vi "UHR-Fleezers Control (fpga) - Leonardo 04-2018.vi"() -> ()   [LabVIEW 2013]
doc: "UHR-Fleezers Instrument Control Code (fpga)"
uses:
  <vilib>/Platform/TimedLoop/XDataNode/timing_clust.ctl
  <vilib>/Platform/TimedLoop/XDataNode/nitl_modes.ctl
  <vilib>/Platform/TimedLoop/XDataNode/wakeup.ctl
  <vilib>/rvi/eio/common/nirviEmuTemplateMethod_errors.vi
  <vilib>/rvi/Emulation/niFpgaSctlEmulationGetInTimedLoop.vi
  <vilib>/rvi/Emulation/niFpgaEmulationReportErrorSimple.vi
  <vilib>/rvi/Emulation/niFpgaGetClockAttributes.vi
  <vilib>/rvi/Emulation/niFpgaCriticalErrorInLSC.vi
  <vilib>/rvi/FIFO/Fifo_Resource/nirvififoEmulationReadFpgaImpl.vi
  <vilib>/rvi/DataTransferAndStorage/Container/Common/niFpgaContainerGetUniqueNameForEmu.vi
  <vilib>/rvi/DataTransferAndStorage/Container/Common/niFpgaContainerExecOnDevCompGetState.vi
  <vilib>/rvi/interface/RandomDataEmulation/nirviRandomDataFPGAFIFO.vi
  <vilib>/rvi/interface/RandomDataEmulation/niFpgaRandomDataHandleErrors.vi
  <vilib>/rvi/eio/common/nirviEmuReportErrorAndStop.vi
  <vilib>/rvi/Emulation/niFpgaProcessEmulError.vi
  <vilib>/rvi/FIFO/Fifo_Resource/nirvififoEmulationWriteFpgaImpl.vi
  <vilib>/rvi/Memory/Memory_Emulation/nirvimemoryFastEmulationFpgaImpl.vi
  <instcachedir>/0/nirvimemoryFastEmulationFpgaImpl_5FBAB50466BC4C939F684F8805638BFC.lvgen/nirvimemoryFastEmulationFpgaImpl_5FBAB50466BC4C939F684F8805638BFC_002.vi
  <vilib>/rvi/Memory/Memory_Emulation/niFpgaMemoryEmulationCacheClearOnFirstRun.vi
  <vilib>/rvi/Memory/Memory_Emulation/nirvimemoryEmulationManagerCache_MakeExclusive.vi
  <vilib>/rvi/Memory/Memory_Emulation/niFpgaMemoryEmulationValidateCache.vi
  <vilib>/rvi/Memory/Memory_Emulation/nirvimemoryEmulationManagerCache_ReleaseExclusive.vi
  <vilib>/rvi/Memory/Memory_Emulation/nirvimemoryEmulationManagerCache_InsertValue.vi
  <vilib>/Utility/error.llb/Clear Errors.vi
  <vilib>/rvi/Memory/Memory_Emulation/nirvimemoryEmulationManagerCache_GetValue.vi
  <vilib>/Platform/TimedLoop/XDataNode/XDataNode.xnode
  <vilib>/eio/EIOMethodNode/EIOMethodNode.xnode
  <vilib>/eio/EIONode/EIONode.xnode
  <vilib>/rvi/DataTransferAndStorage/Container/XNode/niFpgaContainer.xnode
  <vilib>/rvi/FIFO/Fifo_Resource/nirvififoEmulationRead.vi
  <vilib>/rvi/FIFO/Fifo_Resource/niFpgaFifoEmulationRefIn.vi
  <vilib>/rvi/interface/RandomDataEmulation/nirviRandomDataFpgaReadWriteTemplate.vi
  <vilib>/rvi/FIFO/Fifo_Resource/nirvififoEmulationWrite.vi
  <vilib>/rvi/Memory/Memory_Emulation/niFpgaMemoryEmulationRefIn.vi
  <vilib>/addons/control/pid/fpga.llb/XNode/niFpgaPID.xnode
  <vilib>/Platform/TimedLoop/XDataNode/XDNodeRunTimeDep.lvlib
panel:
  in  "Tab Control 2":T1(tab)
  out "BD1 amplitude 1 out":u16
  out "BD1 amplitude 2 out":u16
  in  "FB output range":cluster{"output low":i16, "output high":i16}={"output low"=0, "output high"=3000}
  in  "FB Gains":T2={"proportional gain (Kc)"=10, "integral gain (Kc*Ts/Ti)"=5, "derivative gain (Kc*Td/Ts)"=0}
  in  "RF synth green feedback max":i16=4000
  in  "RD":bool=TRUE
  in  "Swap F1 and F2":bool
  in  "Cont. Scan":bool
  in  "Abort scan":bool
  in  "Cycles per step":u64
  in  "Scan BD":bool
  in  "Number of scans":u16
  in  "Scan steps":u64
  in  "Scan freq.  increment":i64
  out "Scanning":bool
  in  "Start scan":bool
  in  "OSK Bd 1":bool
  in  "Reset Bd 1":bool
  in  "PMODE":bool=TRUE
  in  "Number Interlace Cycles":u8=2 min=1 max=3
  in  "Interlace Off Parameters":u8=1 min=1 max=3
  in  "Interlace ON/OFF":bool
  out "DIO Relative phase":i16
  in  "Phase count adjustment (DIO)":i16
  in  "+ phase (DIO)":bool
  out "DIO Late Counter":u8
  in  "DIO count 1 (ticks)":u16=400
  in  "DIO count 2 (ticks)":u16=400
  in  "DIO count 3 (ticks)":u16=400
  out "AI2 Y Sum Set 2":i16
  out "AI2 Y Sum Set 1":i16
  in  "FB Setpoint Set 1":i16 min=0 step=1
  in  "FB Reset Set 1":bool
  in  "FB On/Off Set 1":bool
  in  "FB Reset Set 2":bool
  in  "FB On/Off Set 2":bool
  in  "FB Setpoint Set 2":i16 min=0 step=1
  out "Scan I":u64
  in  "Amp switch delay":u8=5
  in  "RF synth bd controls green":bool
  in  "Phase Trap 2":fxp<+,14,14>
  in  "Phase Trap 1":fxp<+,14,14>
  in  "Phase offset method":u8
  in  "BD 2 Amplitude 1":u16
  in  "BD 1 Amplitude 1":u16
  in  "BD 2 Frequency 1":u64
  in  "BD 1 Frequency 1":u64
  in  "BD 2 Amplitude 2":u16
  in  "BD 1 Amplitude 2":u16
  in  "BD 2 Frequency 2":u64
  in  "BD 1 Frequency 2":u64
  in  "BD 2 Amplitude 3":u16
  in  "BD 1 Amplitude 3":u16
  in  "BD 2 Frequency 3":u64
  in  "BD 1 Frequency 3":u64
  in  "BD 2 Delay (Ticks)":u8 caption="Count(Ticks)"
  in  "Next trap write delay (ticks)":u8 caption="Count(Ticks)"
  out "Random phase generated":fxp<+,14,14>
  in  "RF phase reset before cycles":bool
  in  "Trap 1 osc enable":bool
  in  "N trap osc periods":i16
  in  "Trap osc period (pts)":i16
  in  "Osc traps":bool
  in  "Initiate trap osc":bool
  in  "Ready Write":bool
  in  "Data":i64
  in  "Address 2":u32
  in  "Osc trap cont.":bool
  in  "Trap 2 osc enable":bool
  out "green FB running":bool
  in  "APD 2 AO scale factor":i16=1
  in  "BD 1 Delay (ticks)":u8
  in  "Tab Control":T3(tab)=enum."MCL trap control"
  in  "Set 3":bool
  in  "Set 2":bool=TRUE
  in  "Set 1":bool=TRUE
  in  "Trap Pos to FIFO":bool
  in  "N of AI1 Int Acq Sets":i16=2 min=1 max=3 step=1
  out "AI Late Counter":u8
  in  "ai count":u16=400
  in  "+ phase":bool
  in  "Phase count adjustment":i16
  out "Relative phase":i16
  in  "AI to FIFO":bool
  out "BD1 Frequency Out 1":u64
  out "BD1 Frequency Out 2":u64
  out "Trap Pos FIFO Timeout":u16
  out "Trap AI FIFO Timeout":u16
  in  "Trap FIFO Set Timeout":i32
  in  "FB Min frequency":u64
  in  "FB Max Frequency":u64
  in  "Dynamic Force FB (Ronen)":bool
  in  "Trap pos. FB Range":T4={"FB2 output low"=-1.0, "FB2 output high"=0.999969482421875}
  in  "Trap Pos. FB Gains":T5={"proportional gain (Kc)"=0.999969482421875, "integral gain (Kc*Ts/Ti)"=0.999969482421875, "derivative gain (Kc*Td/Ts)"=0.0}
  in  "B factor":fxp<+/-,32,16>
  in  "Negate Diff?":bool
  in  "Diff FB Measurement?":bool
  in  "FB Trig Integrate":u32=1
  out "TTrig?":bool
  in  "TTrig Negate Pos":bool=TRUE
  out "Trap Pos FB Int Signal":fxp<+/-,24,9> format="%.18g"
  out "Trap Pos FB Int-Norm Signal":fxp<+/-,16,1> format="%.16g"
  in  "FPGA TTrig Thresh":i64
  in  "FPGA Trap Trig":bool
  out "Trap Pos FB Action":i64
  in  "Trap Pos. FB Offset Factor":i64
  in  "Trap Pos. FB Mult Factor":i64=2
  in  "Trap Pos. FB Reset":bool
  in  "Trap Pos FB Monitor T1 or T2":bool
  in  "AI1 X Scale":u16
  in  "Trap Pos FB Int Count":u16=100
  in  "Trap Pos FB Negate Action":bool
  out "AI1 X Set 2":fxp<+/-,16,1>
  out "AI1 X Set 1":fxp<+/-,16,1>
  in  "Trap Pos. FB SP":fxp<+/-,16,1>
  in  "Force feedback":bool
  out "TTrig Sig":i64
  out "TTrig Fin Thresh":i64
  in  "1D or 2D Scan?":bool
  in  "Abort scan (MCL)":bool
  in  "MCL Scan Axis":bool
  in  "Cont. Scan (MCL)":bool
  out "Scan I (MCL)":u64
  in  "Number of scans (MCL)":u16
  out "Scanning MCL":bool
  in  "Scan steps (MCL)":u64
  in  "Cycles per step (MCL)":u64
  in  "Scan freq.  increment (MCL)":i16
  in  "Start scan (MCL)":bool
  in  "AO2 (X)":i16
  in  "AO1 (Y)":i16
  out "MCL Late Counter":u8
  in  "MCL count":u32=800
  out "MCL Relative Phase":i16
  in  "Phase count adjustment (MCL)":i16
  in  "+ phase (MCL)":bool
  in  "Lifetime events to read blue":u16=100
  in  "Lifetime read blue fifo":bool
  out "lifetime events in fifo":u16
  out "APD2 int gate":bool
  in  "APD Gate Operating Mode":u8 max=2 step=1
  in  "Invert APD Gate":bool
  in  "APD Gate OFF Count":u16=100
  in  "APD Gate ON Count":u16=300
  out "APD 1 Gate Late Counter":u8
  out "APD 1 Gate Relative Phase":i16
  in  "Phase count adjustment (APD 1 Gate)":i16
  in  "+ phase (APD 1 Gate)":bool
  out "APD 2 Counts 0":u32
  out "APD 2 Counts 1":u32
  out "APD 1 Counts 0":u32
  out "APD 1 Counts 1":u32
  in  "Phase count adjustment (APD 2 Gate)":i16
  out "APD 2 Gate Late Counter":u8
  out "APD 2 Gate Relative Phase":i16
  in  "+ phase (APD 2 Gate)":bool
  out "APD 3 Counts 0":u32
  out "APD 3 Counts 1":u32
  out "APD 3 Gate Late Counter":u8
  in  "Phase count adjustment (APD 3 Gate)":i16
  out "APD 3 Gate Relative Phase":i16
  in  "+ phase (APD 3 Gate)":bool
  out "APD1 int gate":bool
  out "APD3 int gate":bool
  in  "Lifetime timeout APD1":u16=200
  in  "APD to FIFO":bool
  in  "APD Acq Rate Count":u32=20000000
  out "APD Acq Late Counter":u16
  out "APD Acq Relative Phase":i16
  in  "+ phase (APD Acq)":bool
  in  "Phase Count Adjustment (APD Acq)":i16
  in  "APD 1 AO scale factor":i16=1
  out "APD2 out state":bool
  out "APD1 out state":bool
  out "APD Acq Late?":bool
  in  "D3 2":i16
  in  "I3 2":i16=5
  in  "P3 2":i16=10
  in  "Green FB Setpoint 2":i16=250 min=0 step=1
  in  "Green FB Reset 2":bool
  in  "Green Filter Flipper":bool
  in  "Green interlace OFF count":u16=100
  out "GI Relative phase":i16
  in  "Phase count adjustment (GI)":i16
  in  "+ phase (GI)":bool
  in  "Green interlace ON count":u16=300
  out "GI Late Counter":u8
  in  "Invert GI":bool
  in  "Operating Mode":u8 max=2 step=1
  in  "Current Out":u16=30000
  in  "Green int current ON count adj":u32=150
  in  "Green interlace OFF count":u32=900
  in  "Green interlace ON count":u32=300
  out "GI Late Counter":u16
  in  "Green FB Count":u32=1200
  in  "Phase count adjustment (GI)":i16=20
  in  "Green FB Setpoint":i16=250 min=0 step=1
  in  "Invert GI":bool
  out "GI Relative phase":i16
  in  "+ phase (GI)":bool
  in  "Phase count adjustment (Green FB)":i16=10
  out "Green Late Counter":u16
  out "Green FB Relative Phase":i16
  in  "+ phase (Green FB)":bool
  out "Green FB Signals":T6
  out "Green FB Sum":i16
  in  "Green FB Gains":T2={"proportional gain (Kc)"=10, "integral gain (Kc*Ts/Ti)"=5, "derivative gain (Kc*Td/Ts)"=0}
  in  "Green FB On/Off":bool
  in  "Green FB Reset":bool
  out "Green FB Late?":bool
  out "GI Late?":bool
  in  "Operating Mode 2":u8=2 max=2 step=1
  in  "+ phase (RI)":bool
  out "RI Relative phase":i16
  out "RI Late Counter":u8
  in  "Red interlace ON count":u16=300
  in  "Red interlace OFF count":u16=100
  in  "Invert RI":bool
  in  "Red Laser Operating Mode":u8 max=2 step=1
  in  "Phase count adjustment (RI)":i16
  in  "Phase count adjustment (BI D)":i16
  in  "Blue Laser Operating Mode (D)":u8 max=2 step=1
  in  "Invert BI (D)":bool
  in  "Blue interlace OFF count (D)":u16=100
  in  "Blue interlace ON count (D)":u16=300
  out "Blue Late Counter (D)":u8
  out "BI Relative phase (D)":i16
  in  "+ phase (BI D)":bool
  in  "Lifetime to FIFO":bool
  out "lifetime (ticks)":u16
  # "Raster Scan AOD"
  # "1 (X)"
  # "2 (Y)"
  # "IR Intensity Feedback (RF BD 1)"
  # "FB Gains Set 1"
  # "FB output range 1"
  # "IR Intensity Feedback (RF BD 2) -\nonly when using BD 2 for green laser AOM (not trap Y)"
  # "Keep below 4096 (12 bits) to stay within range of RF board. Going over doesn't saturate, it truncates higher bits."
  # "RF phase offset control"
  # "Methods are:\n0 - Default, do nothing at all (no phase offset writes)\n1 - Manual phase adjustment\n2 - Cycle the phase adjustment using the input phase numbers as increment values for each cycle"
  # "False is usual, True is external loop method"
  # "Parameters if using the external RF switching loop"
  # "Parameters if using the usual internal RF switching method"
  # "FB Triggering Excitation Laser"
  # "Trap Pos. FB Gains"
  # "Trap Pos. FB Range"
  # "AO1 (Y)"
  # "2D"
  # "Trap 3"
  # "1D"
  # "AO2 (X)"
  # "Fl Laser"
  # "APD AO for aligning"
  # "Detection Loop"
  # "Green fluorescent laser digital gate interlacing loop"
  # "0 Forced ON\n1 Forced OFF\n2 Interlacing"
  # "ALEX settings:"
  # "Controls for usual IA ME controls green AOM"
  # "Controls for RF synth board controls green AOM"
  # "Green FB Gains"
  # "Red fluorescent laser digital gate interlacing loop"
  # "Detection Loop"
  # "0 Forced ON\n1 Forced OFF\n2 Interlacing"
  # "Analog/FB Control Loop\n(Disabled)"
  # "Digital Control Loop"
  # "Blue laser intensity reading"
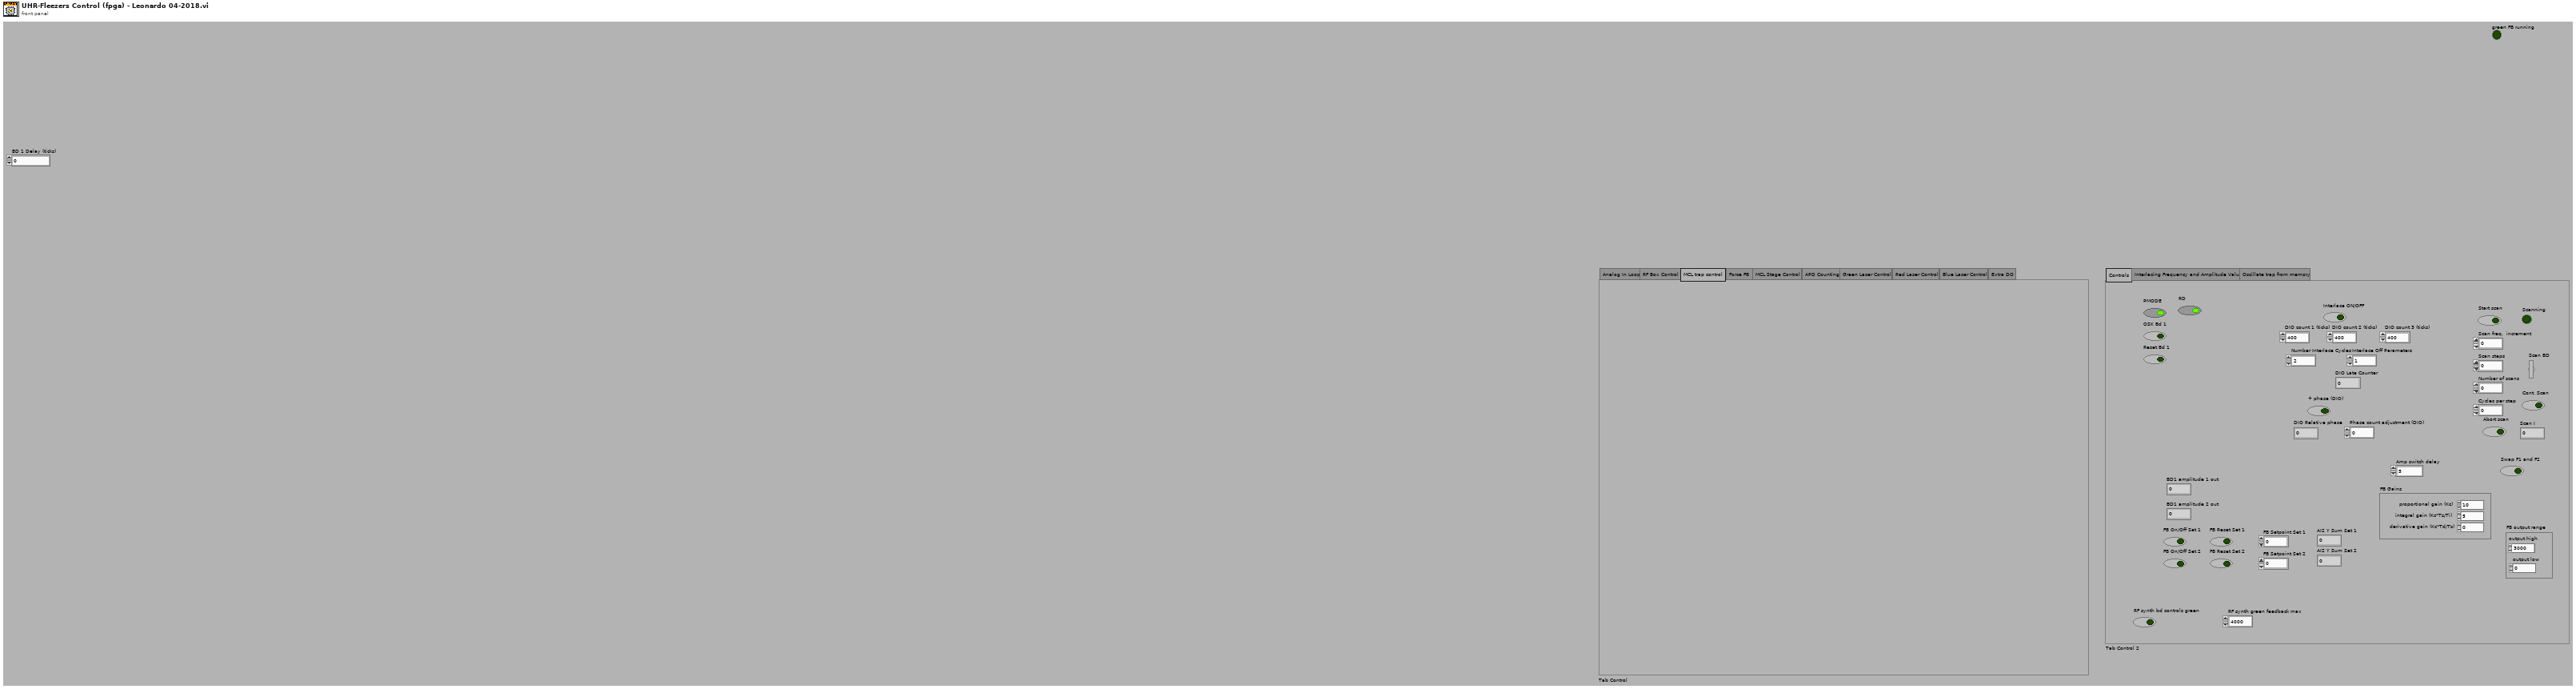
[diagram p1: front panel]
types:
  T1 = enum32{"Controls", "Interlacing Frequency and Amplitude Values", "Oscillate trap from memory"}
  T2 = cluster{"proportional gain (Kc)":i16, "integral gain (Kc*Ts/Ti)":i16, "derivative gain (Kc*Td/Ts)":i16}
  T3 = enum32{"Analog In Loop", "RF Box Control", "MCL trap control", "Force FB", "MCL Stage Control", "APD Counting", "Green Laser Control", "Red Laser Control", "Blue Laser Control", "Extra DO"}
  T4 = cluster{"FB2 output low":fxp<+/-,16,1>, "FB2 output high":fxp<+/-,16,1>}
  T5 = cluster{"proportional gain (Kc)":fxp<+/-,16,1>, "integral gain (Kc*Ts/Ti)":fxp<+/-,16,1>, "derivative gain (Kc*Td/Ts)":fxp<+/-,16,1>}
  T6 = cluster{"Green FB Ch 0":i16, "Green FB Ch 1":i16, "Green FB Ch 2":i16}
  T7 = typedef "XDNodeRunTimeDep.lvlib/timing_clust.ctl" = cluster{"Expected End [f-1]":u64, "Actual End [f-1]":u64, "Finished Late? [f-1]":bool, "Expected End [i-1]":u64, "Actual End [i-1]":u64, "Finished Late? [i-1]":bool, "Expected Start [i]":u64, "Actual Start [i]":u64, "Expected Start [f]":u64, "Actual Start [f]":u64, "Source Name":string, "Structure Name":string, "Period":i64, "Deadline":i64, "Offset":i64, "Start":i64, "Priority":i32, "Timeout":i32, "Mode":T8, "Wakeup Reason":T9, "Error":errorcluster, "Source Type":string, "Secondary Source Type":string, "Global End Time":u64, "Global Start Time":u64, "Frame Duration":u64, "Iteration Duration":u64, "Assigned CPU":i32, "I/O Scan Engine Mode":u32}
  T8 = typedef "XDNodeRunTimeDep.lvlib/nitl_modes.ctl" = enum32{"No Change", "Process missed periods, maintain original phase", "Discard missed periods, maintain original phase", "Process missed periods, ignore original phase", "Discard missed periods, ignore original phase"}
  T9 = typedef "XDNodeRunTimeDep.lvlib/wakeup.ctl" = enum32{"Normal", "Aborted", "Asynchronous wakeup", "Timing source error", "Timed loop error", "Timeout"}
  T10 = cluster{"Chassis2/Mod2/AI0":i16, "Chassis2/Mod2/AI1":i16, "Chassis2/Mod2/AI2":i16}
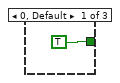
[diagram p3: hidden frame]
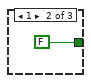
[diagram p4: hidden frame]
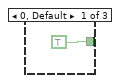
[diagram p8: hidden frame]
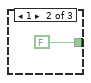
[diagram p9: hidden frame]
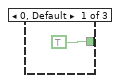
[diagram p10: hidden frame]
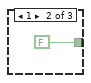
[diagram p11: hidden frame]
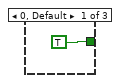
[diagram p13: hidden frame]
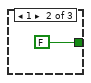
[diagram p14: hidden frame]
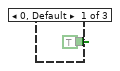
[diagram p15: hidden frame]
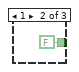
[diagram p16: hidden frame]
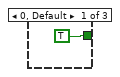
[diagram p18: hidden frame]
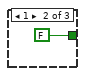
[diagram p19: hidden frame]
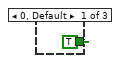
[diagram p20: hidden frame]
diagram:
  w3 = FALSE
  w4 = FALSE
  # "BD2 amp"
  # "BD1 amp"
  # "BD2 amp"
  # "BD1 amp"
  # "timing array current index"
  # "timing array"
  # "timing counter (phase adjusted here)"
  # "late counter"
  n1 = disable-structure shown="Disabled" {
    frame Disabled {
      w14 = i16 2 items=["UnSet Ready", "ReadWrite", "Wait Ready"]
      n2 = while "Handshake memory transfer for trap oscillation sin wave data" {
        shift-right: [w16] -> _
        shift-left: w14 -> [w17]
        stop <- FALSE stop-if-true
        # "Write"
        n3 = case shown="1" w17 {
          tunnel: [w20 w25 w26] -> w16
          frame 3, Default {
            w18 = i16 2 items=["UnSet Ready", "ReadWrite", "Wait Ready"]
            w19 = i16 1 items=["UnSet Ready", "ReadWrite", "Wait Ready"]
            n4 = Select(t=w19, s="Ready Write", f=w18) -> (s? t:f=w20:i16)
          }
          frame 1 {
            w25 = i16 0 items=["UnSet Ready", "ReadWrite", "Wait Ready"]
            n5 = xnode ("Memory Write")("Address"="Address 2", "Data"="Data", "Memory In"=refnum<k21> "Trap osc memory") -> ()  [unwired: 1 out]
          }
          frame 0 {
            w26 = i16 2 items=["UnSet Ready", "ReadWrite", "Wait Ready"]
            n6 = local write "Ready Write"(FALSE ("Ready Read")) -> ()
          }
        }
      }
    }
    frame Enabled {
    }
  }
  n7 = flat-sequence "FPGA initialization to do before running any of the loops" {
    tunnel: [u16 0 ("DIO count 3 (ticks)")] -> w2
    tunnel: [w35] -> _
    frame #0 {
      # "UDCLK out enable and set low"
      # "WR"
      # "BD 2"
      # "BD 1"
      # "With the RF synth board initialization now done in a separate fpga vi, now when this vi is started, board is already configured and is ready for interlacing. Just need to set WR high and enabled UDCLK as write and set to low.\nbefore setting data and address bits."
      # "Start up expansion chassis early\nto avoid delays later"
      # "Set data and address values to something safe (a correct setting) so any initial WR and udclk flipping doesn't have a chance to mess anything up. Safe would be setting an unused data entry:"
      n8 = xnode "FPGA I/O Method Node"("Enable"=TRUE) -> ("FPGA I/O Out"=w29:refnum<k21>)  [unwired: 1 in]
      n9 = xnode "FPGA I/O Method Node"("Enable"=TRUE) -> ("FPGA I/O Out"=w32:refnum<k21>)  [unwired: 1 in]
      n10 = xnode "FPGA I/O Node"("Chassis2/Mod1/AO0"=u16 0 ("Chassis2/Mod4/AO0")) -> ("Chassis2/Mod2/AI0"=w35:i16)  [unwired: 2 in, 2 out]
      n11 = xnode "FPGA I/O Node"("Connector1/DIO15"=TRUE) -> ()  [unwired: 1 in, 1 out]
      n12 = xnode "FPGA I/O Node"("I/O Item"=FALSE ("Connector1/DIO30"), "FPGA I/O In"=w29) -> ()  [unwired: 1 out]
      n13 = xnode "FPGA I/O Node"("I/O Item"=FALSE ("Connector1/DIO30"), "FPGA I/O In"=w32) -> ()  [unwired: 1 out]
      n14 = xnode "FPGA I/O Node"("Connector1/DIO0"=FALSE, "Connector1/DIO1"=FALSE, "Connector1/DIO2"=FALSE, "Connector1/DIO3"=FALSE, "Connector1/DIO4"=FALSE, "Connector1/DIO5"=FALSE, "Connector1/DIO6"=FALSE, "Connector1/DIO7"=FALSE, "Connector1/DIO8"=FALSE, "Connector1/DIO9"=FALSE, "Connector1/DIO10"=FALSE, "Connector1/DIO11"=FALSE, "Connector1/DIO12"=FALSE, "Connector1/DIO13"=FALSE, "Connector1/DIO20"=FALSE, "Connector1/DIO21"=FALSE, "Connector1/DIO22"=FALSE, "Connector1/DIO23"=FALSE, "Connector1/DIO24"=FALSE, "Connector1/DIO25"=FALSE, "Connector1/DIO26"=FALSE, "Connector1/DIO27"=FALSE, "Connector1/DIO14"=FALSE) -> ()  [unwired: 23 in, 23 out]
    }
  }
  n15 = node-c288() -> (w10:T7)  [unwired: 1 in]
  n16 = timed-loop "RF box board DIO control: control bits" {
    timing: w10 -> [_]
    timing-out: [_] -> w9
    tunnel: [w63] -> _
    tunnel: w2 -> [w63]
    stop <- FALSE stop-if-true
    n17 = xnode "FPGA I/O Node"("Connector1/DIO16"="RD", "Connector1/DIO17"="PMODE", "Connector1/DIO18"="OSK Bd 1", "Connector1/DIO19"="Reset Bd 1", "Connector0/DIO3"="Green Filter Flipper") -> ()  [unwired: 5 in, 5 out]
  }
  n18 = node-c288(w9) -> ()
  n19 = local read "AO1 (Y)"() -> (w12:i16)
  n20 = local read "AO2 (X)"() -> (w11:i16)
  n21 = To Unsigned Long Integer(number=w2) -> (unsigned 32bit integer=w5:u32)
  n22 = while "DAQ AI set 1" {
    shift-right: [w70] -> _
    shift-left: w2 -> [w75]
    stop <- FALSE stop-if-true
    n23 = flat-sequence {
      tunnel: w75 -> [w86]
      tunnel: [w85] -> w73
      tunnel: [w86] -> w72
      tunnel: [w96] -> w83
      tunnel: [w95] -> w82
      tunnel: [w94] -> w81
      tunnel: [w93] -> w80
      tunnel: [w92] -> w79
      tunnel: [w91] -> w78
      tunnel: [w90] -> w77
      tunnel: [w89] -> w76
      tunnel: [w88] -> w74
      tunnel: w73 -> [w88]
      tunnel: w72 -> [w87]
      tunnel: [w87] -> w71
      tunnel: [w126] -> w70
      tunnel: w83 -> [w152]
      tunnel: w82 -> [w118]
      tunnel: w81 -> [w119]
      tunnel: w80 -> [w98]
      tunnel: w79 -> [w142]
      tunnel: w78 -> [w141]
      tunnel: w77 -> [w140]
      tunnel: w76 -> [w139]
      tunnel: w74 -> [w136]
      tunnel: w71 -> [w133]
      frame #0 {
        n24 = call "Loop Timer"("Count(Ticks)"=w86) -> ("Tick Count(Ticks)"=w85:u32)
      }
      frame #1 {
        n25 = xnode "FPGA I/O Node"("Connector1/DIO31"=TRUE ("Connector1/DIO33")) -> ("Connector0/AI0"=w96:i16, "Connector0/AI1"=w95:i16, "Connector0/AI2"=w94:i16, "Connector0/AI3"=w93:i16, "Connector0/AI4"=w92:i16, "Connector0/AI5"=w91:i16, "Connector0/AI6"=w90:i16, "Connector0/AI7"=w89:i16)  [unwired: 9 in, 9 out]
      }
      frame #2 {
        w122 = FALSE ("AI to FIFO")
        # "Normalize by trap bead QPD sum, AI3"
        # "Adjust phase after data acquired if button pressed"
        n26 = feedback #1(i16 1) -> (w145:i16)
        n27 = Increment(x=w145) -> (x+1=w151:i16)
        n28 = Scale By Power Of 2(n="AI1 X Scale", x=w118) -> (x*2^n=w116:i16)
        n29 = Greater?(x=w151, y="N of AI1 Int Acq Sets") -> (0:w148:bool)
        n30 = Select(t=i16 1, s=w148, f=w151) -> (s? t:f=w150:i16)
        n31 = feedback-in #1(w150) -> ()
        n32 = Divide(x=w116, y=w98) -> (x/y=w115:fxp<+/-,16,1>)
        n33 = feedback #2(w122) -> (w120:bool)
        n34 = feedback #3(w122) -> (w138:bool)
        n35 = case shown="1, Default" w145 {
          tunnel: w119 -> [w175 w182 _]
          tunnel: ["Set 1" "Set 2" "Set 3"] -> w143
          tunnel: ["AI to FIFO" w184 w189] -> w137
          tunnel: w138 -> [_ w184 w189]
          tunnel: ["Trap Pos to FIFO" w183 w188] -> w121
          tunnel: w120 -> [_ w183 w188]
          tunnel: w115 -> [w174 w181 _]
          tunnel: [w173 w179 FALSE] -> w102
          tunnel: [w172 w180 u64 0 ("BD1 Frequency Out 2")] -> w101
          frame 1, Default {
            n36 = local read "BD1 Frequency Out 1"() -> (w172:u64)
            n37 = Compound Arithmetic op=AND("Trap Pos to FIFO", "Set 1", "AI to FIFO") -> (w173:bool)
            "AI2 Y Sum Set 1" <- w175
            "AI1 X Set 1" <- w174
          }
          frame 2 {
            n38 = local read "BD1 Frequency Out 2"() -> (w180:u64)
            n39 = Compound Arithmetic op=AND(w183, "Set 2", w184) -> (w179:bool)
            "AI2 Y Sum Set 2" <- w182
            "AI1 X Set 2" <- w181
          }
          frame 3 {
          }
        }
        n40 = And(x=w143, y=w137) -> (x .and. y?=w144:bool)
        n41 = case shown="True" w144 {
          tunnel: w152 -> [_ w203]
          tunnel: w118 -> [_ w202]
          tunnel: w119 -> [_ w201]
          tunnel: w98 -> [_ w200]
          tunnel: w142 -> [_ w199]
          tunnel: w141 -> [_ w198]
          tunnel: w140 -> [_ w197]
          tunnel: w139 -> [_ w196]
          tunnel: 0 ("DMA buffer timeout") -> [_ w205]
          frame False {
          }
          frame True {
            n42 = Build Array(w203, w202, w201, w200, w199, w198, w197, w196) -> (w204:i16[])
            n43 = for {
              tunnel: w204 -> [w207] mode=indexing
              tunnel: w205 -> [w208]
              tunnel: [w206] -> w194 mode=indexing
              n44 = xnode ("FIFO Write")("Element"=w207, "Timeout"=w208) -> ("Timed Out?"=w206:bool)  [unwired: 1 in, 1 out]
            }
            n45 = Or Array Elements(Boolean array=w194) -> (logical OR=w191:bool)
            n46 = Boolean To (0,1)(Boolean=w191) -> (0, 1=w193:i16)
            n47 = feedback #4(u16 0) -> (w192:u16)
            n48 = Add(x=w193, y=w192) -> (x+y=w190:u16)
            "Trap AI FIFO Timeout" <- w190
            n49 = feedback-in #4(w190) -> ()
          }
        }
        n50 = feedback-in #2(w121) -> ()
        n51 = feedback-in #3(w137) -> ()
        n52 = case shown="True" w102 {
          tunnel: w101 -> [_ w158]
          tunnel: [u8 0 w155] -> w100
          frame False {
          }
          frame True {
            n53 = Split Number(x=w158) -> (hi(x)=w159:u32, lo(x)=w160:u32)
            n54 = Split Number(x=w159) -> (lo(x)=w161:u16)  [unwired: 1 out]
            n55 = Split Number(x=w160) -> (hi(x)=w162:u16, lo(x)=w163:u16)
            n56 = Build Array "BD 1 nu Stack"(w161, w162, w163) -> (w157:u16[])
            n57 = for {
              tunnel: w157 -> [w170] mode=indexing
              shift-right: [w166] -> w155
              shift-left: u8 0 -> [w167]
              n58 = xnode ("FIFO Method Node")("Element"=w170, "Timeout"="Trap FIFO Set Timeout") -> ("Timed Out?"=w169:bool)  [unwired: 1 in, 1 out]
              n59 = Boolean To (0,1)(Boolean=w169) -> (0, 1=w168:i16)
              n60 = To Unsigned Byte Integer(number=w168) -> (unsigned 8bit integer=w165:u8)
              n61 = Add(x=w165, y=w167) -> (x+y=w166:u8)
            }
          }
        }
        n62 = To Unsigned Word Integer(number=w100) -> (unsigned 16bit integer=w99:u16)
        n63 = feedback #5(u16 0) -> (w113:u16)
        n64 = Add(x=w99, y=w113) -> (x+y=w112:u16)
        "Trap Pos FIFO Timeout" <- w112
        n65 = feedback-in #5(w112) -> ()
        n66 = feedback-in #6(w136) -> ()
        n67 = feedback #6(w136) -> (w135:u32)
        n68 = Subtract(x=w136, y=w135) -> (x-y=w134:u32)
        n69 = xnode "FPGA I/O Node"("Connector1/DIO31"=FALSE ("Connector1/DIO34")) -> ()  [unwired: 1 in, 1 out]
        n70 = Subtract(x=w134, y=w133) -> (x-y=w104:u32)
        n71 = Boolean To (0,1)(Boolean="+ phase") -> (0, 1=w129:i16)
        n72 = Multiply(x=w129, y="Phase count adjustment") -> (x*y=w123:i16)
        n73 = Subtract(x="ai count", y=w104) -> (x-y=w127:u32)
        n74 = Number To Boolean Array(number=w104) -> (Boolean array=w105:bool[])
        n75 = feedback #7(i16 0) -> (w125:i16)
        n76 = Add(x=w127, y=w123) -> (x+y=w126:u32)
        n77 = Subtract(x=w125, y=w123) -> (x-y=w124:i16)
        "Relative phase" <- w124
        n78 = feedback-in #7(w124) -> ()
        n79 = Or Array Elements(Boolean array=w105) -> (logical OR=w103:bool)
        n80 = Boolean To (0,1)(Boolean=w103) -> (0, 1=w110:i16)
        n81 = To Unsigned Byte Integer(number=w110) -> (unsigned 8bit integer=w107:u8)
        n82 = feedback #8(u8 0) -> (w108:u8)
        n83 = Add(x=w107, y=w108) -> (x+y=w106:u8)
        "AI Late Counter" <- w106
        n84 = feedback-in #8(w106) -> ()
      }
    }
  }
  n85 = while "MCL stage control" {
    shift-right: [w221] -> _
    shift-left: w2 -> [w224]
    shift-right: [w214] -> _
    shift-left: w12 -> [w211]
    shift-right: [w213] -> _
    shift-left: w11 -> [w209]
    stop <- FALSE stop-if-true
    n86 = flat-sequence {
      tunnel: w224 -> [w227]
      tunnel: [w226] -> w220
      tunnel: [w227] -> w218
      tunnel: [w229] -> w212
      tunnel: w211 -> [w229]
      tunnel: [w228] -> w210
      tunnel: w209 -> [w228]
      tunnel: w220 -> [w233]
      tunnel: [w233] -> w219
      tunnel: w218 -> [w232]
      tunnel: [w232] -> w217
      tunnel: w212 -> [w231]
      tunnel: w210 -> [w230]
      tunnel: w219 -> [w241]
      tunnel: w217 -> [w240]
      tunnel: [w241] -> w223
      tunnel: [w240] -> w222
      tunnel: [w239] -> w216
      tunnel: [w238] -> w215
      tunnel: [w313] -> w221
      tunnel: w223 -> [w320]
      tunnel: w222 -> [w317]
      tunnel: w216 -> [w315]
      tunnel: w215 -> [w314]
      tunnel: [w315] -> w214
      tunnel: [w314] -> w213
      frame #0 {
        n87 = call "Loop Timer3"("Count(Ticks)"=w227) -> ("Tick Count(Ticks)"=w226:u32)
      }
      frame #1 {
        n88 = xnode "FPGA I/O Node"("Connector0/AO1"=w231, "Connector0/AO2"=w230) -> ()  [unwired: 2 in, 2 out]
      }
      frame #2 {
        n89 = local read "Scanning MCL"() -> (w253:bool)
        n90 = Or(x=w253, y="Start scan (MCL)") -> (x .or. y?=w248:bool)
        n91 = Not(x="Abort scan (MCL)") -> (.not. x?=w246:bool)
        n92 = And(x=w246, y=w248) -> (x .and. y?=w245:bool)
        n93 = case "Raster scan" shown="False" w245 {
          tunnel: [w254 w297] -> w250
          tunnel: "Start scan (MCL)" -> [_ w282]
          tunnel: [w254 w258] -> w234
          frame False {
            w254 = i16 0
            n94 = local write "Scanning MCL"(FALSE ("scanning")) -> ()
          }
          frame True {
            w268 = i16 0
            w267 = u64 0
            # "scan incr."
            # "freq. incr. mult."
            # "count steps"
            # "count number of cycles"
            n95 = feedback #9(w267) -> (w294:u64)
            n96 = Select(t=w267, s=w282, f=w294) -> (s? t:f=w296:u64)
            n97 = Increment(x=w296) -> (x+1=w293:u64)
            n98 = Greater?(x="Cycles per step (MCL)", y=w293) -> (0:w277:bool)
            n99 = Select(t=w293, s=w277, f=w267) -> (s? t:f=w292:u64)
            n100 = feedback-in #9(w292) -> ()
            n101 = feedback #10(w267) -> (w291:u64)
            n102 = Select(t=w267, s=w282, f=w291) -> (s? t:f=w286:u64)
            n103 = Increment(x=w286) -> (x+1=w290:u64)
            n104 = Add(x="Scan steps (MCL)", y="Scan steps (MCL)") -> (x+y=w289:u64)
            n105 = Select(t=w286, s=w277, f=w290) -> (s? t:f=w272:u64)
            n106 = Greater?(x=w289, y=w272) -> (0:w271:bool)
            n107 = Select(t=w272, s=w271, f=w267) -> (s? t:f=w287:u64)
            n108 = feedback-in #10(w287) -> ()
            n109 = Equal?(x="Scan steps (MCL)", y=w272) -> (x = y?=w276:bool)
            n110 = Greater?(x="Scan steps (MCL)", y=w286) -> (0:w285:bool)
            n111 = feedback #11(w268) -> (w288:i16)
            n112 = Select(t=w268, s=w282, f=w288) -> (s? t:f=w274:i16)
            n113 = Increment(x=w274) -> (x+1=w284:i16)
            n114 = Decrement(x=w274) -> (x-1=w283:i16)
            n115 = Select(t=w284, s=w285, f=w283) -> (s? t:f=w275:i16)
            n116 = Select(t=w274, s=w276, f=w275) -> (s? t:f=w273:i16)
            n117 = Select(t=w274, s=w277, f=w273) -> (s? t:f=w269:i16)
            n118 = Select(t=w269, s=w271, f=w268) -> (s? t:f=w270:i16)
            n119 = feedback-in #11(w270) -> ()
            n120 = feedback #12(w267) -> (w281:u64)
            n121 = Select(t=w267, s=w282, f=w281) -> (s? t:f=w256:u64)
            n122 = Increment(x=w256) -> (x+1=w278:u64)
            n123 = Select(t=w256, s=w271, f=w278) -> (s? t:f=w257:u64)
            n124 = Greater?(x="Number of scans (MCL)", y=w257) -> (0:w264:bool)
            n125 = Multiply(x="Scan freq.  increment (MCL)", y=w274) -> (x*y=w297:i16)
            n126 = Select(t=TRUE, s="Cont. Scan (MCL)", f=w264) -> (s? t:f=w263:bool)
            "Scanning MCL" <- w263
            n127 = Select(t=w257, s=w263, f=w267) -> (s? t:f=w279:u64)
            n128 = feedback-in #12(w279) -> ()
            n129 = Increment(x=w257) -> (x+1=→"Scan I (MCL)":u64)
            n130 = To Word Integer(number=w256) -> (16bit integer=w259:i16)
            n131 = Multiply(x=w259, y="Scan freq.  increment (MCL)") -> (x*y=w258:i16)
          }
        }
        n132 = Select(t=w234, s="1D or 2D Scan?", f=i16 0) -> (s? t:f=w235:i16)
        n133 = Select(t=w250, s="MCL Scan Axis", f=w235) -> (s? t:f=w251:i16)
        n134 = Select(t=w235, s="MCL Scan Axis", f=w250) -> (s? t:f=w249:i16)
        n135 = Add(x="AO2 (X)", y=w249) -> (x+y=w238:i16)
        n136 = Add(x="AO1 (Y)", y=w251) -> (x+y=w239:i16)
      }
      frame #3 {
        n137 = feedback-in #13(w320) -> ()
        n138 = feedback #13(w320) -> (w319:u32)
        n139 = Boolean To (0,1)(Boolean="+ phase (MCL)") -> (0, 1=w311:i16)
        n140 = Subtract(x=w320, y=w319) -> (x-y=w318:u32)
        n141 = Multiply(x=w311, y="Phase count adjustment (MCL)") -> (x*y=w307:i16)
        n142 = Subtract(x=w318, y=w317) -> (x-y=w299:u32)
        n143 = Subtract(x="MCL count", y=w299) -> (x-y=w309:u32)
        n144 = feedback #14(i16 0) -> (w308:i16)
        n145 = Subtract(x=w308, y=w307) -> (x-y=w306:i16)
        "MCL Relative Phase" <- w306
        n146 = feedback-in #14(w306) -> ()
        n147 = Number To Boolean Array(number=w299) -> (Boolean array=w300:bool[])
        n148 = Or Array Elements(Boolean array=w300) -> (logical OR=w298:bool)
        n149 = Boolean To (0,1)(Boolean=w298) -> (0, 1=w305:i16)
        n150 = Add(x=w309, y=w307) -> (x+y=w313:u32)
        n151 = To Unsigned Byte Integer(number=w305) -> (unsigned 8bit integer=w302:u8)
        n152 = feedback #15(u8 0) -> (w303:u8)
        n153 = Add(x=w302, y=w303) -> (x+y=w301:u8)
        "MCL Late Counter" <- w301
        n154 = feedback-in #15(w301) -> ()
      }
    }
  }
  n155 = while "Trap RF control, main calculations (raster scanning, intensity and position feedback, phase control etc) with primary timing trigger" {
    shift-right: [w336] -> _
    shift-left: w2 -> [w335]
    shift-right: [w334] -> _
    shift-left: FALSE ("Swap F1 and F2") -> [w333]
    shift-right: [w329] -> _
    shift-left: u16 0 ("BD 1 Amplitude 3") -> [w326]
    shift-right: [w328] -> _
    shift-left: u16 0 ("BD 2 Amplitude 3") -> [w324]
    shift-right: [w323] -> _
    shift-left: u64 0 -> [w322]
    stop <- FALSE stop-if-true
    n156 = flat-sequence {
      tunnel: w333 -> [w342]
      tunnel: w335 -> [w339]
      tunnel: [w342] -> w332
      tunnel: [w338] -> w331
      tunnel: [w339] -> w330
      tunnel: [w341] -> w327
      tunnel: w326 -> [w341]
      tunnel: [w340] -> w325
      tunnel: w324 -> [w340]
      tunnel: [w353] -> w336
      tunnel: [w352] -> w334
      tunnel: w332 -> [w351]
      tunnel: w331 -> [w350]
      tunnel: w330 -> [w349]
      tunnel: [w348] -> w329
      tunnel: [w347] -> w328
      tunnel: w327 -> [w346]
      tunnel: w325 -> [w345]
      tunnel: [w344] -> w323
      tunnel: w322 -> [w343]
      frame #0 {
        n157 = call "Loop Timer2"("Count(Ticks)"=w339) -> ("Tick Count(Ticks)"=w338:u32)
      }
      frame #1 {
        n158 = flat-sequence {
          tunnel: w351 -> [w361]
          tunnel: w346 -> [w355]
          tunnel: w345 -> [w354]
          tunnel: [w423] -> w353
          tunnel: [w435] -> w352
          tunnel: w350 -> [w429]
          tunnel: w349 -> [w426]
          tunnel: [w372] -> w348
          tunnel: [w371] -> w347
          tunnel: [w363] -> w344
          tunnel: w343 -> [w362]
          frame #0 {
            w356 = -1 ("Timeout")
            # "Operation when you need a long delay for either X or Y to synchonize AOD light out phase (> ~100 ticks)\nor want shorter trap ON timing. Puts some of the delay timing in parallel with the later computations."
            # "Trigger the external loop by sending the boolean FSK value through a FIFO.\nTiming is precise."
            n159 = Boolean To (0,1)(Boolean=w361) -> (0, 1=w360:i16)
            n160 = To Unsigned Word Integer(number=w360) -> (unsigned 16bit integer=w359:u16)
            n161 = xnode ("FIFO Method Node")("Element"=w359, "Timeout"=w356) -> ("FIFO Out"=w358:refnum<k21>)  [unwired: 1 in, 1 out]
            n162 = xnode ("FIFO Method Node")("Element"=w355, "Timeout"=w356, "FIFO In"=w358) -> ("FIFO Out"=w357:refnum<k21>)  [unwired: 1 out]
            n163 = xnode ("FIFO Method Node")("Element"=w354, "Timeout"=w356, "FIFO In"=w357) -> ()  [unwired: 2 out]
          }
          frame #1 {
            # "Just counts, wraps around, 8 bit"
            # "Which trap cycle"
            # "Only save the 3rd set's amp in the loop"
            # "If this is NOT set 3 AND NOT (RF synth controls green AND green FB running)\nthen use this sets amp value (otherwise keep the green feedback value)"
            # "Just flips back and forth."
            # "If interlacing is off, this is which cycle to use."
            # "Keep track of trap cycles (trap 1, 2, 3...)"
            # "This is the prior cycle's on time"
            # "increment timing\nindex, reset to 0 if \nend of matrix"
            # "Reset to begginning (1) when number of cycles reached."
            # "timing index"
            # "build byte stacks for writing data\n(must correspond to addresses array constant)"
            # "Timing housekeeping"
            # "Adjust phase if late\n(maintains constant phase relationship between cycles)"
            n164 = feedback #16(u8 0 ("t")) -> (w432:u8)
            n165 = Increment(x=w432) -> (x+1=w471:u8)
            n166 = Increment(x="Number Interlace Cycles") -> (x+1=w466:u8)
            n167 = Equal?(x=w471, y=w466) -> (x = y?=w473:bool)
            n168 = Select(t=u8 1, s=w473, f=w471) -> (s? t:f=w431:u8)
            n169 = feedback-in #16(w431) -> ()
            n170 = Increment(x=w431) -> (x+1=w468:u8)
            n171 = Equal?(x=w468, y=w466) -> (x = y?=w469:bool)
            n172 = Select "This cycle"(t=u8 1, s=w469, f=w468) -> (s? t:f=w465:u8)
            n173 = Select(t=w465, s="Interlace ON/OFF", f="Interlace Off Parameters") -> (s? t:f=w382:u8)
            n174 = feedback-in #17(w429) -> ()
            n175 = feedback #17(w429) -> (w428:u32)
            n176 = Select(t=w431, s="Interlace ON/OFF", f="Interlace Off Parameters") -> (s? t:f=w464:u8)
            n177 = Subtract(x=w429, y=w428) -> (x-y=w427:u32)
            n178 = Subtract "The error"(x=w427, y=w426) -> (x-y=w410:u32)
            n179 = case shown="1, Default" w464 {
              tunnel: ["DIO count 1 (ticks)" "DIO count 2 (ticks)" "DIO count 3 (ticks)"] -> w425
              frame 1, Default {
              }
              frame 2 {
              }
              frame 3 {
              }
            }
            n180 = Number To Boolean Array(number=w410) -> (Boolean array=w411:bool[])
            n181 = Or Array Elements(Boolean array=w411) -> (logical OR=w409:bool)
            n182 = Boolean To (0,1)(Boolean=w409) -> (0, 1=w416:i16)
            n183 = To Unsigned Byte Integer(number=w416) -> (unsigned 8bit integer=w413:u8)
            n184 = feedback #18(u8 0) -> (w414:u8)
            n185 = Add(x=w413, y=w414) -> (x+y=w412:u8)
            "DIO Late Counter" <- w412
            n186 = feedback-in #18(w412) -> ()
            n187 = Subtract(x=w425, y=w410) -> (x-y=w424:u32)
            n188 = local read "green FB running"() -> (w395:bool)
            n189 = And(x=w395, y="RF synth bd controls green") -> (x .and. y?=w394:bool)
            n190 = feedback #19(i64 0 ("y")) -> (w407:i64)
            n191 = case "Synchronize trap oscillations - always begin/end with trap 1" shown="1, Default" w382 {
              tunnel: [w579 w580 w581] -> w408
              tunnel: w407 -> [w579 w580 _]
              frame 2 {
              }
              frame 3 {
              }
              frame 1, Default {
                n192 = Or(x="Osc traps", y="Initiate trap osc") -> (x .or. y?=w583:bool)
                n193 = case "Trap sine oscillation (or whatever pattern is stored in memory)" shown="True" w583 {
                  tunnel: [i64 0 ("y") w587] -> w581
                  tunnel: "Initiate trap osc" -> [_ w590]
                  frame False {
                  }
                  frame True {
                    w594 = u16 0
                    w592 = -1
                    n194 = local write "Initiate trap osc"(FALSE ("Initiate trap osc")) -> ()
                    n195 = feedback #20(w594) -> (w596:u16)
                    n196 = Select(t=w594, s=w590, f=w596) -> (s? t:f=w595:u16)
                    n197 = Greater Or Equal?(x=w595, y="Trap osc period (pts)") -> (x >= y?=w601:bool)
                    n198 = Or(x=w590, y=w601) -> (x .or. y?=w602:bool)
                    n199 = Select(t=u16 0, s=w602, f=w595) -> (s? t:f=w586:u16)
                    n200 = feedback #21(w592) -> (w593:i32)
                    n201 = Select(t=w592, s=w590, f=w593) -> (s? t:f=w591:i32)
                    n202 = Increment(x=w591) -> (x+1=w598:i32)
                    n203 = Equal?(x=w586, y=u16 0) -> (x = y?=w599:bool)
                    n204 = Increment(x=w586) -> (x+1=w606:u16)
                    n205 = feedback-in #20(w606) -> ()
                    n206 = Select(t=w598, s=w599, f=w591) -> (s? t:f=w597:i32)
                    n207 = feedback-in #21(w597) -> ()
                    n208 = case shown="False" "Osc trap cont." {
                      tunnel: w597 -> [w610 _]
                      frame False {
                        n209 = Greater Or Equal?(x=w610, y="N trap osc periods") -> (x >= y?=w608:bool)
                        n210 = Not(x=w608) -> (.not. x?=w607:bool)
                        n211 = local write "Osc traps"(w607) -> ()
                      }
                      frame True {
                      }
                    }
                    n212 = xnode ("Memory Read")("Address"=w586, "Memory In"=refnum<k21> "Trap osc memory") -> ("Data"=w587:i64)  [unwired: 1 out]
                  }
                }
              }
            }
            n213 = case shown="1, Default" w382 {
              tunnel: [w624 w839 "BD 1 Frequency 3"] -> w461
              tunnel: [w674 w838 w864] -> w398
              tunnel: ["BD 2 Amplitude 1" "BD 2 Amplitude 2" w863] -> w390
              tunnel: [w621 w835 "BD 1 Amplitude 3"] -> w372
              tunnel: "FB Gains" -> [w644 w845 _]
              tunnel: "FB output range" -> [w645 w844 _]
              tunnel: w408 -> [w642 w842 _]
              tunnel: "BD 2 Frequency 1" -> [w639 _ _]
              tunnel: "BD 2 Frequency 2" -> [_ w838 _]
              tunnel: "BD 2 Frequency 3" -> [_ _ w864]
              tunnel: w394 -> [_ _ w862]
              tunnel: [w624 w836 w857] -> w363
              tunnel: w362 -> [w623 w836 w857]
              frame 1, Default {
                w659 = fxp<+/-,24,9> 0.0 ("AI1 X Set 2")
                w653 = u16 0
                w671 = u64 0 ("f")
                # "Changed by Ronen - correction \nby PID is now implemented not on \nthe Base BD1 frequency but on the last\nfrequency sent."
                # "Added by Ronen -\nUpper and Lower \nLimits for the FB \ngenerated frequency\nto avoid losing bead \nwhen tether breaks"
                # "Explanation of raster scanning:\n1. Cycles: increment counter by 1 every time interlace cycle returns to trap 1. As long as \n  Cycle per Step is larger than counter, keep incrementing counter and do not change step counter.\n  Once counter is equal to Cycles per step, zero counter and increment step counter.\n2. Steps: Increments up every time cycles counter equals cycles per step. Performs the following:\n- To determine DIRECTION of frequency change:  If ScanstepX2 is EQUAL to step counter (full for-back scan finished)\n   frequency increment is set to zero, AND step counter is set to zero. \n   Otherwise: if no change to step counter (because cycleperstep>cycle counter), then no change to frequency\n   increment. \n   If step counter has changed (cycleperstep=cycle counter), then need to figure out direction of frequency change:\n   if step counter is EQUAL to Scansteps: No change to frequency increment\n   Otherwise: If scan steps > step counter - 1 (forward scan NOT completed): increment frequency by 1\n                       If scan steps equal or smaller than step counter -1 (forward scan completed): increment frequency by -1\n\n3. Scans: Increment scan counter every time step counter equals 2Xscan steps (full for-back scan completed)\n    if number of scans > scan counter: Send TRUE to scanning, continue scan\n    if number of scans = scan counter: Send FALSE to Scanning, Scan finished.\n\n  The wire with the asterik can be used as the index for getting the mirror positions in the offset scan."
                # "This signal integration happens no matter what\nso that correct setpoints can be chosen before \nturning on the FB."
                # "Trap 1"
                n214 = local read "AI1 X Set 2"() -> (w636:fxp<+/-,16,1>)
                n215 = local read "AI1 X Set 1"() -> (w656:fxp<+/-,16,1>)
                n216 = local read "Scanning"() -> (w675:bool)
                n217 = Multiply(x=w636, y="B factor") -> (x*y=w634:fxp<+/-,48,17>)
                n218 = Or(x=w675, y="Start scan") -> (x .or. y?=w669:bool)
                n219 = case shown="True" "Diff FB Measurement?" {
                  tunnel: w634 -> [w692 w701]
                  tunnel: w656 -> [w691 w702]
                  tunnel: [w689 w693] -> w657
                  frame False {
                    n220 = Select(t=w691, s="Trap Pos FB Monitor T1 or T2", f=w692) -> (s? t:f=w689:fxp<+/-,48,17>)
                  }
                  frame True {
                    n221 = Subtract(x=w702, y=w701) -> (x-y=w694:fxp<+/-,48,17>)
                    n222 = Not(x="Negate Diff?") -> (.not. x?=w700:bool)
                    n223 = Boolean To (0,1)(Boolean="Negate Diff?") -> (0, 1=w698:i16)
                    n224 = Boolean To (0,1)(Boolean=w700) -> (0, 1=w699:i16)
                    n225 = Negate(x=w698) -> (-x=w697:i16)
                    n226 = Add(x=w697, y=w699) -> (x+y=w695:i16)
                    n227 = Multiply(x=w695, y=w694) -> (x*y=w693:fxp<+/-,63,32>)
                  }
                }
                n228 = Not(x="Abort scan") -> (.not. x?=w667:bool)
                n229 = And(x=w667, y=w669) -> (x .and. y?=w666:bool)
                n230 = case "For raster scanning" shown="True" w666 {
                  tunnel: [u64 0 w825] -> w672
                  tunnel: "Start scan" -> [_ w810]
                  tunnel: [u64 1 w787] -> w637
                  frame False {
                    n231 = local write "Scanning"(FALSE ("scanning")) -> ()
                  }
                  frame True {
                    w794 = i64 0
                    w793 = u64 0
                    # "scan incr."
                    # "freq. incr. mult."
                    # "count steps"
                    # "count number of cycles"
                    n232 = feedback #22(w793) -> (w822:u64)
                    n233 = Select(t=w793, s=w810, f=w822) -> (s? t:f=w824:u64)
                    n234 = Increment(x=w824) -> (x+1=w821:u64)
                    n235 = Greater?(x="Cycles per step", y=w821) -> (0:w803:bool)
                    n236 = Select(t=w821, s=w803, f=w793) -> (s? t:f=w820:u64)
                    n237 = feedback-in #22(w820) -> ()
                    n238 = feedback #23(w793) -> (w819:u64)
                    n239 = Select(t=w793, s=w810, f=w819) -> (s? t:f=w814:u64)
                    n240 = Increment(x=w814) -> (x+1=w818:u64)
                    n241 = Add(x="Scan steps", y="Scan steps") -> (x+y=w817:u64)
                    n242 = Select(t=w814, s=w803, f=w818) -> (s? t:f=w798:u64)
                    n243 = Greater?(x=w817, y=w798) -> (0:w797:bool)
                    n244 = Select(t=w798, s=w797, f=w793) -> (s? t:f=w815:u64)
                    n245 = feedback-in #23(w815) -> ()
                    n246 = Equal?(x="Scan steps", y=w798) -> (x = y?=w802:bool)
                    n247 = Greater?(x="Scan steps", y=w814) -> (0:w813:bool)
                    n248 = feedback #24(w794) -> (w816:i64)
                    n249 = Select(t=w794, s=w810, f=w816) -> (s? t:f=w800:i64)
                    n250 = Increment(x=w800) -> (x+1=w812:i64)
                    n251 = Decrement(x=w800) -> (x-1=w811:i64)
                    n252 = Select(t=w812, s=w813, f=w811) -> (s? t:f=w801:i64)
                    n253 = Select(t=w800, s=w802, f=w801) -> (s? t:f=w799:i64)
                    n254 = Select(t=w800, s=w803, f=w799) -> (s? t:f=w795:i64)
                    n255 = Select(t=w795, s=w797, f=w794) -> (s? t:f=w796:i64)
                    n256 = feedback-in #24(w796) -> ()
                    n257 = feedback #25(w793) -> (w809:u64)
                    n258 = Select(t=w793, s=w810, f=w809) -> (s? t:f=w805:u64)
                    n259 = Increment(x=w805) -> (x+1=w806:u64)
                    n260 = Select(t=w805, s=w797, f=w806) -> (s? t:f=w804:u64)
                    n261 = Greater?(x="Number of scans", y=w804) -> (0:w790:bool)
                    n262 = Multiply(x="Scan freq.  increment", y=w800) -> (x*y=w825:i64)
                    n263 = Select(t=TRUE, s="Cont. Scan", f=w790) -> (s? t:f=w789:bool)
                    "Scanning" <- w789
                    n264 = Select(t=w804, s=w789, f=w793) -> (s? t:f=w807:u64)
                    n265 = feedback-in #25(w807) -> ()
                    n266 = Increment(x=w804) -> (x+1=w787:u64)
                  }
                }
                "Scan I" <- w637
                n267 = feedback #26(w653) -> (w652:u16)
                n268 = Increment(x=w652) -> (x+1=w654:u16)
                n269 = Greater Or Equal?(x=w654, y="Trap Pos FB Int Count") -> (x >= y?=w622:bool)
                n270 = Select(t=w653, s=w622, f=w654) -> (s? t:f=w655:u16)
                n271 = feedback-in #26(w655) -> ()
                n272 = feedback #27(w659) -> (w658:fxp<+/-,24,9>)
                n273 = Add(x=w657, y=w658) -> (x+y=w651:fxp<+/-,24,9>)
                n274 = case "Trap 1 X intensity feedback" shown="True" "FB On/Off Set 1" {
                  tunnel: "BD 1 Amplitude 1" -> [w827 _]
                  tunnel: [w827 w831] -> w621
                  tunnel: w645 -> [_ w828]
                  tunnel: w644 -> [_ w829]
                  frame False {
                  }
                  frame True {
                    n275 = local read "AI2 Y Sum Set 1"() -> (w832:i16)
                    n276 = call "Slower PID.vi"("process variable"=w832, "reset?"="FB Reset Set 1", "setpoint"="FB Setpoint Set 1", "PID gains (x 2^8)"=w829, "output range"=w828) -> ("output"=w833:i16)  [unwired: 10 out]
                    n277 = To Unsigned Word Integer(number=w833) -> (unsigned 16bit integer=w831:u16)
                  }
                }
                "BD1 amplitude 1 out" <- w621
                n278 = Select(t=w659, s=w622, f=w651) -> (s? t:f=w662:fxp<+/-,24,9>)
                n279 = feedback-in #27(w662) -> ()
                n280 = Divide(x=w651, y="Trap Pos FB Int Count") -> (x/y=w646:fxp<+/-,16,1>)
                n281 = feedback #28(fxp<+/-,24,9> 0.0 ("AI1 X Set 2")) -> (w663:fxp<+/-,24,9>)
                n282 = Select(t=w651, s=w622, f=w663) -> (s? t:f=w664:fxp<+/-,24,9>)
                "Trap Pos FB Int Signal" <- w664
                n283 = feedback-in #28(w664) -> ()
                n284 = feedback #29(fxp<+/-,16,1> 0.0 ("Trap Pos FB Int-Norm Signal")) -> (w648:fxp<+/-,16,1>)
                n285 = Select(t=w646, s=w622, f=w648) -> (s? t:f=w647:fxp<+/-,16,1>)
                "Trap Pos FB Int-Norm Signal" <- w647
                n286 = feedback-in #29(w647) -> ()
                n287 = case "For position feedback" shown="True" "Force feedback" {
                  tunnel: [i64 0 w708] -> w629
                  tunnel: w646 -> [_ w705]
                  tunnel: w622 -> [_ w704]
                  frame False {
                  }
                  frame True {
                    n288 = feedback #30(i64 0) -> (w707:i64)
                    n289 = case shown="True" w704 {
                      tunnel: [w709 w713] -> w708
                      tunnel: w707 -> [w709 _]
                      tunnel: w705 -> [_ w712]
                      frame False {
                      }
                      frame True {
                        n290 = xnode ("PID")("process variable"=w712, "reset?"="Trap Pos. FB Reset", "setpoint"="Trap Pos. FB SP", "PID gains"="Trap Pos. FB Gains", "output range"="Trap pos. FB Range") -> ("output"=w722:fxp<+/-,16,1>)
                        n291 = Negate(x=w722) -> (-x=w721:fxp<+/-,17,2>)
                        n292 = Select(t=w721, s="Trap Pos FB Negate Action", f=w722) -> (s? t:f=w718:fxp<+/-,17,2>)
                        n293 = Scale By Power Of 2(n=u32 15, x=u32 1) -> (x*2^n=w715:u32)
                        n294 = Multiply(x=w718, y=w715) -> (x*y=w714:fxp<+/-,17,17>)
                        n295 = To Quad Integer(1:w714) -> (0:w726:i64)
                        "Trap Pos FB Action" <- w726
                        n296 = Multiply(x=w726, y="Trap Pos. FB Mult Factor") -> (x*y=w724:i64)
                        n297 = Add(x=w724, y="Trap Pos. FB Offset Factor") -> (x+y=w713:i64)
                        n298 = disable-structure shown="Disabled" {
                          disable-tunnel: w713 -> [w733 _]
                          frame Disabled {
                            w737 = u32 0
                            n299 = feedback #31() -> (w734:i64)  [unwired: 1 in]
                            n300 = Add(x=w733, y=w734) -> (x+y=w731:i64)
                            n301 = feedback #32(w737) -> (w739:u32)
                            n302 = Increment(x=w739) -> (x+1=w728:u32)
                            n303 = Greater Or Equal?(x=w728, y="FB Trig Integrate") -> (x >= y?=w729:bool)
                            n304 = Select(t=i64 0, s=w729, f=w731) -> (s? t:f=w735:i64)
                            n305 = feedback-in #31(w735) -> ()
                            n306 = Select(t=w737, s=w729, f=w728) -> (s? t:f=w738:u32)
                            n307 = feedback-in #32(w738) -> ()
                            n308 = And(x=w729, y="FPGA Trap Trig") -> (x .and. y?=w736:bool)
                            n309 = case "Trap FB trigger excitation laser ON" shown="True" w736 {
                              tunnel: w731 -> [_ w743]
                              tunnel: w728 -> [_ w741]
                              frame False {
                              }
                              frame True {
                                n310 = Not(x="TTrig Negate Pos") -> (.not. x?=w750:bool)
                                n311 = Boolean To (0,1)(Boolean="TTrig Negate Pos") -> (0, 1=w748:i16)
                                n312 = Boolean To (0,1)(Boolean=w750) -> (0, 1=w749:i16)
                                n313 = Negate(x=w748) -> (-x=w747:i16)
                                n314 = Add(x=w747, y=w749) -> (x+y=w746:i16)
                                n315 = Multiply(x=w746, y=w743) -> (x*y=w745:i64)
                                "TTrig Sig" <- w745
                                n316 = Multiply(x="FPGA TTrig Thresh", y=w741) -> (x*y=w742:i64)
                                "TTrig Fin Thresh" <- w742
                                n317 = Greater Or Equal?(x=w745, y=w742) -> (x >= y?=w744:bool)
                                n318 = case shown="True" w744 {
                                frame False {
                                }
                                frame True {
                                w753 = TRUE ("Green FB On/Off")
                                w755 = u8 2 ("Operating Mode")
                                n319 = local write "Operating Mode"(w755) -> ()
                                n320 = local write item#-1(w755) -> ()
                                n321 = local write item#-1(w753) -> ()
                                n322 = local write "FPGA Trap Trig"(FALSE ("FPGA Trap Trig")) -> ()
                                "TTrig?" <- w753
                                }
                                }
                              }
                            }
                          }
                          frame Enabled {
                          }
                        }
                      }
                    }
                    n323 = feedback-in #30(w708) -> ()
                  }
                }
                n324 = And(x="Force feedback", y="Dynamic Force FB (Ronen)") -> (x .and. y?=w631:bool)
                n325 = case shown="True" w631 {
                  tunnel: w629 -> [w680 w684]
                  tunnel: [w679 w683] -> w630
                  tunnel: w623 -> [_ w682]
                  tunnel: w622 -> [_ w681]
                  frame False {
                    # "(BD1 Frequency 1)"
                    n326 = Add(x="BD 1 Frequency 1", y=w680) -> (x+y=w679:u64)
                  }
                  frame True {
                    n327 = case shown="True" w681 {
                      tunnel: w684 -> [_ w688]
                      tunnel: [w685 w687] -> w683
                      tunnel: w682 -> [w685 w686]
                      frame False {
                      }
                      frame True {
                        n328 = Add(x=w686, y=w688) -> (x+y=w687:u64)
                      }
                    }
                  }
                }
                n329 = Select(t=w642, s="Trap 1 osc enable", f=i64 0) -> (s? t:f=w640:i64)
                n330 = Select(t=w671, s="Scan BD", f=w672) -> (s? t:f=w670:u64)
                n331 = Select(t=w672, s="Scan BD", f=w671) -> (s? t:f=w628:u64)
                n332 = Add(x=w670, y=w639) -> (x+y=w674:u64)
                n333 = Compound Arithmetic op=ADD(w640, w630, w628) -> (w627:u64)
                n334 = In Range and Coerce(upper limit="FB Max Frequency", x=w627, lower limit="FB Min frequency") -> (coerced(x)=w624:u64)  [unwired: 1 out]
                "BD1 Frequency Out 1" <- w624
              }
              frame 2 {
                # "Trap 2"
                n335 = case "Trap 2 X intensity feedback" shown="True" "FB On/Off Set 2" {
                  tunnel: [w849 w852] -> w835
                  tunnel: "BD 1 Amplitude 2" -> [w849 _]
                  tunnel: w845 -> [_ w851]
                  tunnel: w844 -> [_ w850]
                  frame False {
                  }
                  frame True {
                    n336 = local read "AI2 Y Sum Set 2"() -> (w855:i16)
                    n337 = call "Slower PID.vi"("process variable"=w855, "reset?"="FB Reset Set 2", "setpoint"="FB Setpoint Set 2", "PID gains (x 2^8)"=w851, "output range"=w850) -> ("output"=w853:i16)  [unwired: 10 out]
                    n338 = To Unsigned Word Integer(number=w853) -> (unsigned 16bit integer=w852:u16)
                  }
                }
                "BD1 amplitude 2 out" <- w835
                n339 = Select(t=w842, s="Trap 2 osc enable", f=i64 0) -> (s? t:f=w841:i64)
                n340 = Add(x="BD 1 Frequency 2", y=w841) -> (x+y=w839:u64)
                "BD1 Frequency Out 2" <- w839
              }
              frame 3 {
                # "Remember if FB was previously on/off"
                # "Fluorescence period"
                n341 = feedback #33(FALSE) -> (w858:bool)
                n342 = case shown="True" w862 {
                  tunnel: [w868 w884] -> w863
                  tunnel: "BD 2 Amplitude 3" -> [w868 _]
                  tunnel: [FALSE TRUE] -> w859
                  tunnel: w858 -> [_ w870]
                  frame False {
                  }
                  frame True {
                    # "Makes it so first time FB run when turned on, the PID sees the detector intensity from the last time FB was running, rather than something near zero. Especially assuming the setpoint is not changing, this will make the FB more stable when resuming, and not overshoot the turnon intensity."
                    # "FB output range: 0 should be low, full scale is 12 bits.\nBut be careful not to go over, then higher bits just get ignored by RF board, so output will actually jump down and be unstable. Keep it under 4000 to be safe."
                    n343 = local read "Green FB Sum"() -> (w869:i16)
                    n344 = feedback-in #34(w869) -> ()
                    n345 = feedback #34(i16 0 ("Green FB Sum")) -> (w872:i16)
                    n346 = Select(t=w869, s=w870, f=w872) -> (s? t:f=w871:i16)
                    n347 = Bundle("P3 2"="P3 2", "I3 2"="I3 2", "D3 2"="D3 2") -> (w883:cluster{"P3 2":i16, "I3 2":i16, "D3 2":i16})  [unwired: 1 in]
                    n348 = Bundle("RF synth green feedback max"="RF synth green feedback max", i16 0) -> (w875:cluster{"RF synth green feedback max":i16, i16})  [unwired: 1 in]
                    n349 = call "Slower PID.vi"("process variable"=w871, "reset?"="Green FB Reset 2", "setpoint"="Green FB Setpoint 2", "PID gains (x 2^8)"=w883, "output range"=w875) -> ("output"=w885:i16)  [unwired: 10 out]
                    n350 = To Unsigned Word Integer(number=w885) -> (unsigned 16bit integer=w884:u16)
                  }
                }
                n351 = feedback-in #33(w859) -> ()
              }
            }
            n352 = feedback-in #19(w408) -> ()
            n353 = Split Number(x=w461) -> (hi(x)=w460:u32, lo(x)=w459:u32)
            n354 = Boolean To (0,1)(Boolean="+ phase (DIO)") -> (0, 1=w421:i16)
            n355 = Split Number(x=w460) -> (lo(x)=w458:u16)  [unwired: 1 out]
            n356 = Split Number(x=w459) -> (hi(x)=w457:u16, lo(x)=w456:u16)
            n357 = Split Number(x=w458) -> (hi(x)=w450:u8, lo(x)=w449:u8)
            n358 = Split Number(x=w457) -> (hi(x)=w448:u8, lo(x)=w447:u8)
            n359 = Split Number(x=w456) -> (hi(x)=w446:u8, lo(x)=w445:u8)
            n360 = Multiply(x=w421, y="Phase count adjustment (DIO)") -> (x*y=w417:i16)
            n361 = feedback #35(TRUE) -> (w404:bool)
            n362 = Not(x=w404) -> (.not. x?=w403:bool)
            n363 = feedback-in #35(w403) -> ()
            n364 = feedback #36(i16 0) -> (w419:i16)
            n365 = Subtract(x=w419, y=w417) -> (x-y=w418:i16)
            "DIO Relative phase" <- w418
            n366 = feedback-in #36(w418) -> ()
            n367 = Add(x=w424, y=w417) -> (x+y=w423:u32)
            n368 = Build Array "BD 1 nu Stack"(w450, w449, w448, w447, w446, w445) -> (w444:u8[])
            n369 = Not Equal?(x=w382, y=u8 3) -> (x != y?=w391:bool)
            n370 = case "Store in RF board F1 or F2" shown="True" w403 {
              tunnel: [w612 w616] -> w435
              tunnel: [u8 10 u8 4] -> w436
              tunnel: "Swap F1 and F2" -> [w613 w616]
              tunnel: "BD 2 Frequency 1" -> [_ w615]
              tunnel: "BD 2 Frequency 2" -> [w611 _]
              tunnel: [w611 w615] -> w399
              frame False {
                # "for RF synth controls\ngreen: F1/F2 stay same"
                # "F2 address (hex)"
                n371 = Not(x=w613) -> (.not. x?=w612:bool)
              }
              frame True {
                # "low chooses F1"
                # "F1 address (hex)"
              }
            }
            n372 = Select(t=w399, s="RF synth bd controls green", f=w398) -> (s? t:f=w397:u64)
            n373 = Split Number(x=w397) -> (hi(x)=w455:u32, lo(x)=w454:u32)
            n374 = Split Number(x=w455) -> (lo(x)=w453:u16)  [unwired: 1 out]
            n375 = Split Number(x=w454) -> (hi(x)=w452:u16, lo(x)=w451:u16)
            n376 = Split Number(x=w453) -> (hi(x)=w443:u8, lo(x)=w442:u8)
            n377 = Split Number(x=w452) -> (hi(x)=w441:u8, lo(x)=w440:u8)
            n378 = Split Number(x=w451) -> (hi(x)=w439:u8, lo(x)=w438:u8)
            n379 = feedback #37(u16 0 ("BD 2 Amplitude 3")) -> (w388:u16)
            n380 = Select(t=w388, s=w391, f=w390) -> (s? t:f=w389:u16)
            n381 = feedback-in #37(w389) -> ()
            n382 = And(x=w391, y=w394) -> (x .and. y?=w393:bool)
            n383 = Build Array "BD 2 nu Stack"(w443, w442, w441, w440, w439, w438) -> (w437:u8[])
            n384 = Select(t=w388, s=w393, f=w390) -> (s? t:f=w371:u16)
            n385 = flat-sequence "Update trap RF synth board settings to be used for the upcoming trap cycle." {
              tunnel: w437 -> [w528]
              tunnel: w444 -> [w529]
              tunnel: [w529] -> w386
              tunnel: [w528] -> w385
              tunnel: w436 -> [w530]
              tunnel: w386 -> [w532]
              tunnel: w385 -> [w531]
              tunnel: w373 -> [w543]
              tunnel: w375 -> [w542]
              tunnel: w374 -> [w541]
              frame #0 {
                # "To possibly delay\nthese writes to very\nend of loop (for x and\ny phase adjust)"
                n386 = call "Wait8"("Count(Ticks)"="Next trap write delay (ticks)") -> ()  [unwired: 1 out]
              }
              frame #1 {
                # "Next trap RF frequency:\n\nWrite next trap cycle frequency to buffer."
                n387 = for {
                  tunnel: w532 -> [w538] mode=indexing
                  tunnel: w531 -> [w537] mode=indexing
                  tunnel: w530 -> [w535]
                  i -> [w536]
                  n388 = To Unsigned Byte Integer(number=w536) -> (unsigned 8bit integer=w533:u8)
                  n389 = Add(x=w535, y=w533) -> (x+y=w534:u8)
                  n390 = call "write to RF synth bd.vi"("Address Byte"=w534, "BD 2 Byte"=w537, "BD 1 Byte"=w538) -> ()
                }
              }
              frame #2 {
                w539 = TRUE ("Connector1/DIO15")
                # "Send udclk high\n(BD 1 and 2) to make the new frequency active in F1 or F2 word. But it won't actually be the used frequency until FSK switches to it (begining of next cycle)."
                n391 = xnode "FPGA I/O Node"("Connector1/DIO30"=w539, "Connector1/DIO29"=w539) -> ()  [unwired: 2 in, 2 out]
              }
              frame #3 {
                w540 = FALSE ("Connector1/DIO15")
                n392 = xnode "FPGA I/O Node"("Connector1/DIO30"=w540, "Connector1/DIO29"=w540) -> ()  [unwired: 2 in, 2 out]
              }
              frame #4 {
                # "Next trap RF phase offset:\n\nSet the next trap cycle amplitude to the buffer. Won't become active until udclk is set high at proper time at the begining of the next cycle."
                n393 = case shown="True" w543 {
                  tunnel: w542 -> [_ w544]
                  tunnel: w541 -> [_ w545]
                  frame False {
                  }
                  frame True {
                    # "phase 1 address start"
                    n394 = for {
                      tunnel: w544 -> [w552] mode=indexing
                      tunnel: w545 -> [w551] mode=indexing
                      tunnel: u8 0 -> [w549]
                      i -> [w550]
                      n395 = To Unsigned Byte Integer(number=w550) -> (unsigned 8bit integer=w547:u8)
                      n396 = Add(x=w549, y=w547) -> (x+y=w548:u8)
                      n397 = call "write to RF synth bd.vi"("Address Byte"=w548, "BD 2 Byte"=w551, "BD 1 Byte"=w552) -> ()
                    }
                  }
                }
              }
              frame #5 {
                # "Prep to reset RF phase to zero at start of next cycle. Only reset BD 1. Do nothing to BD 2. This puts the settings in the buffer. A udclk high will make both this phase reset and possibly a new phase offset setting active."
                n398 = case shown="True" "RF phase reset before cycles" {
                  frame False {
                  }
                  frame True {
                    w555 = u8 66  # BD 1 reset
                    n399 = call "write to RF synth bd.vi"("Address Byte"=u8 31, "BD 2 Byte"=u8 2, "BD 1 Byte"=w555) -> ()
                  }
                }
              }
              frame #6 {
                # "Address"
                # "Data BD 2"
                # "Data BD 1"
                # "If phase reset wasn't chosen previously, these actions will have no affect. For both BD's, data should be binary 10, and address should be hex 1F (bin 01 1111)"
                # "This sets up the digital communication lines to restart phase accumulation (start RF running agin). It cancels out the possible phase reset. Just need to set WR DIO low then udclk DIOhigh  to make this happen. Doing this here early (and not using the usual board write function) speeds things up.\n\nRestarts RF (BD 1 only, BD2 never stopped in first place)."
                n400 = xnode "FPGA I/O Node"("Connector1/DIO0"=FALSE, "Connector1/DIO1"=FALSE, "Connector1/DIO2"=FALSE, "Connector1/DIO3"=FALSE, "Connector1/DIO4"=FALSE, "Connector1/DIO5"=FALSE, "Connector1/DIO6"=TRUE, "Connector1/DIO7"=FALSE, "Connector1/DIO8"=FALSE, "Connector1/DIO9"=TRUE, "Connector1/DIO10"=TRUE, "Connector1/DIO11"=TRUE, "Connector1/DIO12"=TRUE, "Connector1/DIO13"=TRUE, "Connector1/DIO20"=FALSE, "Connector1/DIO21"=FALSE, "Connector1/DIO22"=FALSE, "Connector1/DIO23"=FALSE, "Connector1/DIO24"=FALSE, "Connector1/DIO25"=FALSE, "Connector1/DIO26"=TRUE, "Connector1/DIO27"=FALSE) -> ()  [unwired: 22 in, 22 out]
              }
            }
            n401 = feedback #38(fxp<+,8,8> 0.0) -> (w368:fxp<+,8,8>)
            n402 = Increment(x=w368) -> (x+1=w366:fxp<+,8,8>)
            n403 = feedback-in #38(w366) -> ()
            n404 = case "Trap RF phase offset control methods" shown="3" "Phase offset method" {
              tunnel: [fxp<+,14,14> 0.0 ("Phase BD 1") w478 w493 w522] -> w376
              tunnel: "Phase Trap 1" -> [_ w479 w494 _]
              tunnel: w382 -> [_ w480 w495 w523]
              tunnel: [FALSE TRUE TRUE TRUE] -> w373
              tunnel: "Phase Trap 2" -> [_ w476 w491 _]
              tunnel: w366 -> [_ _ w490 _]
              frame 0, Default {
              }
              frame 1 {
                # "Constant increment of phase offset with each trap cycle. This results in a constant phase difference between trap cycles. \nOnly for traps 1 and 2 (set phase offset to zero for set three)."
                n405 = case shown="1, Default" w480 {
                  tunnel: w479 -> [_ _ w486]
                  tunnel: [w482 fxp<+,14,14> 0.0 w487] -> w478
                  tunnel: w476 -> [w481 _ _]
                  frame 2 {
                    n406 = feedback #39(fxp<+,14,14> 0.0) -> (w484:fxp<+,14,14>)
                    n407 = Add(x=w481, y=w484) -> (x+y=w482:fxp<+,14,14>)
                    n408 = feedback-in #39(w482) -> ()
                  }
                  frame 3 {
                  }
                  frame 1, Default {
                    n409 = feedback #40(fxp<+,14,14> 0.0) -> (w489:fxp<+,14,14>)
                    n410 = Add(x=w486, y=w489) -> (x+y=w487:fxp<+,14,14>)
                    n411 = feedback-in #40(w487) -> ()
                  }
                }
              }
              frame 2 {
                # "Changing increment of phase offset with each trap cycle. This results in a constant change in phase difference between trap cycles. \nOnly for traps 1 and 2 (set phase offset to zero for set three)."
                n412 = case shown="2" w495 {
                  tunnel: w494 -> [_ _ w505]
                  tunnel: [w496 fxp<+,14,14> 0.0 w503] -> w493
                  tunnel: w491 -> [w498 _ _]
                  tunnel: w490 -> [w499 _ w506]
                  frame 2 {
                    n413 = Multiply(x=w498, y=w499) -> (x*y=w497:fxp<+,16,16>)
                    n414 = feedback #41(fxp<+,14,14> 0.0) -> (w501:fxp<+,14,14>)
                    n415 = Add(x=w497, y=w501) -> (x+y=w496:fxp<+,14,14>)
                    n416 = feedback-in #41(w496) -> ()
                  }
                  frame 3 {
                  }
                  frame 1, Default {
                    n417 = Multiply(x=w505, y=w506) -> (x*y=w504:fxp<+,16,16>)
                    n418 = feedback #42(fxp<+,14,14> 0.0) -> (w508:fxp<+,14,14>)
                    n419 = Add(x=w504, y=w508) -> (x+y=w503:fxp<+,14,14>)
                    n420 = feedback-in #42(w503) -> ()
                  }
                }
              }
              frame 3 {
                w515 = u32 1013904223  # LCG constant C (add)
                w517 = fxp<+,21,21> 1664525.0  # LCG constant A (multiply)
                # "Set a random phase offset. Random number generated using the LCG method. Constants and method taken from NI white noise generator code (method is general though)."
                # "shift to 14 significant bits"
                n421 = feedback #43(u32 4294967295 ("seed")) -> (w512:u32)
                n422 = Multiply(x=w512, y=w517) -> (x*y=w516:u32)
                n423 = Split Number(x=w512) -> (hi(x)=w518:u16)  [unwired: 1 out]
                n424 = To Unsigned Word Integer(number=w518) -> (unsigned 16bit integer=w510:u16)
                n425 = Add(x=w516, y=w515) -> (x+y=w514:fxp<+,32,32>)
                n426 = To Unsigned Long Integer(number=w514) -> (unsigned 32bit integer=w511:u32)
                n427 = feedback-in #43(w511) -> ()
                n428 = Scale By Power Of 2(n=i8 -2 ("Uniform scale factor"), x=w510) -> (x*2^n=w519:u16)
                n429 = To Fixed-Point(number=w519) -> (fixed-point=w509:fxp<+,14,14>)  [unwired: 1 in]
                "Random phase generated" <- w509
                n430 = case shown="1, Default" w523 {
                  tunnel: [w524 fxp<+,14,14> 0.0 w526] -> w522
                  tunnel: w509 -> [w524 _ w526]
                  frame 2 {
                  }
                  frame 3 {
                  }
                  frame 1, Default {
                  }
                }
              }
            }
            n431 = To Unsigned Word Integer(number=w376) -> (unsigned 16bit integer=w381:u16)
            n432 = Split Number(x=w381) -> (hi(x)=w379:u8, lo(x)=w380:u8)
            n433 = Split Number(x=u16 0) -> (hi(x)=w377:u8, lo(x)=w378:u8)
            n434 = Build Array ("BD 1 A Stack")(w379, w380) -> (w375:u8[])
            n435 = Build Array ("BD 1 A Stack")(w377, w378) -> (w374:u8[])
          }
        }
      }
    }
  }
  n436 = while "APD 2 Counter" {
    tunnel: w2 -> [_]
    stop <- FALSE stop-if-true
    n437 = flat-sequence {
      frame #0 {
        n438 = xnode "FPGA I/O Method Node"("FPGA I/O In"=refnum<k21> "Connector0/DIO8" ("APD 2 DO"), "Timeout"=-1) -> ()  [unwired: 2 out]
      }
      frame #1 {
        n439 = local read "APD2 int gate"() -> (w889:bool)
        n440 = case shown="True" w889 {
          frame False {
          }
          frame True {
            n441 = local read "APD2 out state"() -> (w890:bool)
            n442 = case shown="True" w890 {
              frame False {
                n443 = local read "APD 2 Counts 0"() -> (w892:u32)
                n444 = Increment(x=w892) -> (x+1=→"APD 2 Counts 0":u32)
              }
              frame True {
                n445 = local read "APD 2 Counts 1"() -> (w894:u32)
                n446 = Increment(x=w894) -> (x+1=→"APD 2 Counts 1":u32)
              }
            }
          }
        }
      }
    }
  }
  n447 = while "Green fluorescent laser interlacing (Current to IA 532 nm AOM ME amp)." {
    shift-right: [w900] -> _
    shift-left: w2 -> [w903]
    shift-right: [w897] -> _
    shift-left: i16 0 -> [w895]
    stop <- FALSE stop-if-true
    n448 = flat-sequence {
      tunnel: w903 -> [w906]
      tunnel: [w907] -> w902
      tunnel: [w906] -> w901
      tunnel: [w905] -> w896
      tunnel: w895 -> [w905]
      tunnel: [w910] -> w899
      tunnel: w902 -> [w910]
      tunnel: [w909] -> w898
      tunnel: w901 -> [w909]
      tunnel: w896 -> [w908]
      tunnel: [w923] -> w900
      tunnel: [w939] -> w897
      tunnel: w899 -> [w952]
      tunnel: w898 -> [w949]
      frame #0 {
        n449 = call "Loop Timer10"("Count(Ticks)"=w906) -> ("Tick Count(Ticks)"=w907:u32)
      }
      frame #1 {
        n450 = xnode "FPGA I/O Node"("Chassis2/Mod1/AO0"=w908) -> ()  [unwired: 1 in, 1 out]
      }
      frame #2 {
        n451 = local read "RF synth bd controls green"() -> (w914:bool)
        n452 = Subtract(x="Green interlace OFF count", y="Green int current ON count adj") -> (x-y=w932:u32)
        n453 = feedback-in #44(w952) -> ()
        n454 = feedback #44(w952) -> (w951:u32)
        n455 = Add(x="Green int current ON count adj", y="Green interlace ON count") -> (x+y=w933:u32)
        n456 = Subtract(x=w952, y=w951) -> (x-y=w950:u32)
        n457 = Subtract(x=w950, y=w949) -> (x-y=w916:u32)
        n458 = Not(x=w914) -> (.not. x?=w912:bool)
        n459 = Number To Boolean Array(number=w916) -> (Boolean array=w917:bool[])
        n460 = Boolean To (0,1)(Boolean="+ phase (GI)") -> (0, 1=w929:i16)
        n461 = Or Array Elements(Boolean array=w917) -> (logical OR=w915:bool)
        "GI Late?" <- w915
        n462 = Boolean To (0,1)(Boolean=w915) -> (0, 1=w922:i16)
        n463 = Multiply(x=w929, y="Phase count adjustment (GI)") -> (x*y=w925:i16)
        n464 = To Unsigned Word Integer(number=w922) -> (unsigned 16bit integer=w918:u16)
        n465 = feedback #45(u16 0) -> (w920:u16)
        n466 = Add(x=w918, y=w920) -> (x+y=w919:u16)
        "GI Late Counter" <- w919
        n467 = feedback-in #45(w919) -> ()
        n468 = feedback #46(i16 0) -> (w926:i16)
        n469 = Subtract(x=w926, y=w925) -> (x-y=w924:i16)
        "GI Relative phase" <- w924
        n470 = feedback-in #46(w924) -> ()
        n471 = feedback #47(TRUE) -> (w944:bool)
        n472 = case shown="2" "Operating Mode 2" {
          tunnel: [TRUE FALSE w969] -> w934
          tunnel: w944 -> [_ _ w966]
          frame 0, Default {
          }
          frame 1 {
          }
          frame 2 {
            n473 = Not(x=w966) -> (.not. x?=w968:bool)
            n474 = Select(t=w968, s="Invert GI", f=w966) -> (s? t:f=w969:bool)
          }
        }
        n475 = And(x=w934, y="Green FB On/Off") -> (x .and. y?=w913:bool)
        "green FB running" <- w913
        n476 = And(x=w913, y=w912) -> (x .and. y?=w911:bool)
        n477 = case shown="True" w911 {
          tunnel: "Current Out" -> [w953 _]
          tunnel: [w953 w958] -> w938
          frame False {
          }
          frame True {
            n478 = local read "Green FB Sum"() -> (w954:i16)
            n479 = call "Slower PID.vi"("process variable"=w954, "reset?"="Green FB Reset", "setpoint"="Green FB Setpoint", "PID gains (x 2^8)"="Green FB Gains", "output range"=cluster{"output high":i16, "output low":i16} {"output high"=32767, "output low"=-32768} ("Green FB output range")) -> ("output"=w962:i16)  [unwired: 10 out]
            n480 = To Long Integer(number=w962) -> (32bit integer=w955:i32)
            n481 = Add(x=w955, y=32768) -> (x+y=w957:i32)
            n482 = To Unsigned Word Integer(number=w957) -> (unsigned 16bit integer=w958:u16)
          }
        }
        n483 = Not(x=w944) -> (.not. x?=w941:bool)
        n484 = Select(t=w933, s=w941, f=w932) -> (s? t:f=w946:u32)
        n485 = Subtract(x=w946, y=w916) -> (x-y=w927:u32)
        n486 = Add(x=w927, y=w925) -> (x+y=w923:u32)
        n487 = feedback-in #47(w941) -> ()
        n488 = Boolean To (0,1)(Boolean=w934) -> (0, 1=w940:i16)
        n489 = To Unsigned Word Integer(number=w940) -> (unsigned 16bit integer=w937:u16)
        n490 = Multiply(x=w937, y=w938) -> (x*y=w939:u16)
      }
    }
  }
  n491 = while "APD 1 Counter" {
    tunnel: w2 -> [_]
    stop <- FALSE stop-if-true
    n492 = flat-sequence {
      frame #0 {
        n493 = xnode "FPGA I/O Method Node"("FPGA I/O In"=refnum<k21> "Connector0/DIO4" ("APD 1 DO"), "Timeout"=-1) -> ()  [unwired: 2 out]
      }
      frame #1 {
        n494 = local read "APD1 int gate"() -> (w973:bool)
        n495 = case shown="False" w973 {
          frame False {
          }
          frame True {
            n496 = local read "APD1 out state"() -> (w974:bool)
            n497 = case shown="True" w974 {
              frame False {
                n498 = local read "APD 1 Counts 0"() -> (w976:u32)
                n499 = Increment(x=w976) -> (x+1=→"APD 1 Counts 0":u32)
              }
              frame True {
                n500 = local read "APD 1 Counts 1"() -> (w978:u32)
                n501 = Increment(x=w978) -> (x+1=→"APD 1 Counts 1":u32)
              }
            }
          }
        }
      }
    }
  }
  n502 = while "RF synth board interlacing timing loop" {
    tunnel: w2 -> [_]
    stop <- FALSE stop-if-true
    # "This loop is stalled until the RF FIFO get a value. With this method we gain additional delay time (because  we allow the rest of the main RF loop to procede while this loop waits to send the switch signals - a form of parallelism). This helps to simplify the main RF code. \n\nThe code also allow optimal interlacing while also controlling trap RF phase. \n\nNote: a lot of work has gone into optimizing these methods and it is unclear how they can be made any faster or better than this (many failed tries). Right now there is essentially ~4 ticks (~90 ns ns) of imperfection in the switching from trap 1 to trap 2. ~2 ticks of no RF (phase reset) then ~2 ticks of trap 2 with the wrong amplitude (T1 amplitude). The total ticks is 200, so not a big error.\n\nPhase can be precisely set for each trap. Phase reset and switching, has similar delays as fsk frequency switching. And phase reset and phase offset changes are also not simultaneous. So we can't perfectly line everything up.\n\nIf you start from amp zero though (as for trap 1), the on switch is perfect. Likewise the off is perfect for trap 2. \n\nThe green laser switching is also perfect because of its reduced duty cycle and delays in fsk switching between 80 and 0 MHz."
    n503 = xnode ("FIFO Read")("Timeout"=-1) -> ("Element"=w1025:u16, "FIFO Out"=w1021:refnum<k21>)  [unwired: 1 in, 1 out]
    n504 = Equal To 0?(x=w1025) -> (x = 0?=w1022:bool)
    n505 = Not(x=w1022) -> (.not. x?=w979:bool)
    n506 = flat-sequence "BD 1 and 2 RF phase and amplitude switching" {
      tunnel: w979 -> [_]
      tunnel: w1014 -> [w1129]
      tunnel: w1013 -> [w1128]
      tunnel: w1012 -> [w1127]
      tunnel: w1011 -> [w1126]
      tunnel: w1010 -> [w1125]
      tunnel: w1009 -> [w1124]
      tunnel: w1008 -> [w1123]
      tunnel: w1007 -> [w1122]
      tunnel: w1005 -> [w1121]
      tunnel: w1004 -> [w1120]
      tunnel: w1003 -> [w1119]
      tunnel: w1001 -> [w1117]
      tunnel: w1000 -> [w1116]
      tunnel: w999 -> [w1115]
      tunnel: w1002 -> [w1118]
      tunnel: w1006 -> [w1114]
      tunnel: w998 -> [w1153]
      tunnel: w997 -> [w1152]
      tunnel: w996 -> [w1151]
      tunnel: w995 -> [w1150]
      tunnel: w994 -> [w1149]
      tunnel: w993 -> [w1148]
      tunnel: w992 -> [w1147]
      tunnel: w991 -> [w1146]
      tunnel: w990 -> [w1145]
      tunnel: w988 -> [w1144]
      tunnel: w987 -> [w1143]
      tunnel: w986 -> [w1142]
      tunnel: w985 -> [w1141]
      tunnel: w984 -> [w1140]
      tunnel: w983 -> [w1139]
      tunnel: w989 -> [w1138]
      frame #0 {
        # "Delay to align amp/frequency switching depending on the method used.\n\nCan also give enough time to do the parallel amplitude calculations"
        n507 = call "Wait2"("Count(Ticks)"="Amp switch delay") -> ()  [unwired: 1 out]
      }
      frame #1 {
        w1109 = TRUE ("Connector1/DIO30")
        # "make phase offset and phase reset active with buffer transfer"
        n508 = xnode "FPGA I/O Node"("Connector1/DIO29"=w1109, "Connector1/DIO30"=w1109) -> ()  [unwired: 2 in, 2 out]
      }
      frame #2 {
        w1110 = FALSE ("Connector1/DIO15")
        # "write phase restart to buffer and reset udclk"
        n509 = xnode "FPGA I/O Node"("Connector1/DIO29"=w1110, "Connector1/DIO30"=w1110, "Connector1/DIO15"=FALSE ("Connector1/DIO14")) -> ()  [unwired: 3 in, 3 out]
      }
      frame #3 {
        w1112 = TRUE ("Connector1/DIO15")
        # "make phase restart active"
        # "reset WR"
        n510 = xnode "FPGA I/O Node"("Connector1/DIO15"=w1112, "Connector1/DIO29"=w1112, "Connector1/DIO30"=w1112) -> ()  [unwired: 3 in, 3 out]
      }
      frame #4 {
        w1113 = FALSE ("Connector1/DIO30")
        # "Address"
        # "set amp byte 1, and reset udclk"
        n511 = xnode "FPGA I/O Node"("Connector1/DIO0"=w1129, "Connector1/DIO1"=w1128, "Connector1/DIO2"=w1127, "Connector1/DIO3"=w1126, "Connector1/DIO4"=w1125, "Connector1/DIO5"=w1124, "Connector1/DIO6"=w1123, "Connector1/DIO7"=w1122, "Connector1/DIO8"=TRUE, "Connector1/DIO9"=FALSE, "Connector1/DIO10"=FALSE, "Connector1/DIO11"=FALSE, "Connector1/DIO12"=FALSE, "Connector1/DIO13"=TRUE, "Connector1/DIO20"=w1114, "Connector1/DIO21"=w1121, "Connector1/DIO22"=w1120, "Connector1/DIO23"=w1119, "Connector1/DIO24"=w1118, "Connector1/DIO25"=w1117, "Connector1/DIO26"=w1116, "Connector1/DIO27"=w1115, "Connector1/DIO30"=w1113, "Connector1/DIO29"=w1113) -> ()  [unwired: 24 in, 24 out]
      }
      frame #5 {
        # "write amp byte 1 to buffer"
        n512 = xnode "FPGA I/O Node"("Connector1/DIO15"=FALSE ("Connector1/DIO14")) -> ()  [unwired: 1 in, 1 out]
      }
      frame #6 {
        # "reset WR"
        n513 = xnode "FPGA I/O Node"("Connector1/DIO15"=TRUE) -> ()  [unwired: 1 in, 1 out]
      }
      frame #7 {
        # "Address"
        # "set amp byte 2"
        n514 = xnode "FPGA I/O Node"("Connector1/DIO0"=w1153, "Connector1/DIO1"=w1152, "Connector1/DIO2"=w1151, "Connector1/DIO3"=w1150, "Connector1/DIO4"=w1149, "Connector1/DIO5"=w1148, "Connector1/DIO6"=w1147, "Connector1/DIO7"=w1146, "Connector1/DIO8"=TRUE, "Connector1/DIO9"=FALSE, "Connector1/DIO10"=FALSE, "Connector1/DIO11"=FALSE, "Connector1/DIO12"=TRUE, "Connector1/DIO13"=FALSE, "Connector1/DIO20"=w1145, "Connector1/DIO21"=w1138, "Connector1/DIO22"=w1144, "Connector1/DIO23"=w1143, "Connector1/DIO24"=w1142, "Connector1/DIO25"=w1141, "Connector1/DIO26"=w1140, "Connector1/DIO27"=w1139) -> ()  [unwired: 22 in, 22 out]
      }
      frame #8 {
        # "write amp byte 2"
        n515 = xnode "FPGA I/O Node"("Connector1/DIO15"=FALSE ("Connector1/DIO14")) -> ()  [unwired: 1 in, 1 out]
      }
      frame #9 {
        w1161 = TRUE ("Connector1/DIO15")
        # "transfer amp bytes 1 and 2 and reset WR"
        n516 = xnode "FPGA I/O Node"("Connector1/DIO29"=w1161, "Connector1/DIO30"=w1161, "Connector1/DIO15"=TRUE ("Connector1/DIO14")) -> ()  [unwired: 3 in, 3 out]
      }
      frame #10 {
        w1163 = FALSE ("Connector1/DIO14")
        # "reset udclk"
        n517 = xnode "FPGA I/O Node"("Connector1/DIO29"=w1163, "Connector1/DIO30"=w1163) -> ()  [unwired: 2 in, 2 out]
      }
    }
    n518 = flat-sequence "FSK BD 1 (trap X)" {
      tunnel: w979 -> [w1027]
      tunnel: [w1027] -> w982
      tunnel: w982 -> [w1028]
      frame #0 {
        n519 = call "Wait"("Count(Ticks)"="BD 1 Delay (ticks)") -> ()  [unwired: 1 out]
      }
      frame #1 {
        # "switch frequency"
        n520 = xnode "FPGA I/O Node"("Connector1/DIO36"=w1028) -> ()  [unwired: 1 in, 1 out]
      }
    }
    n521 = flat-sequence "FSK BD 2 (trap Y or green laser AOM)" {
      tunnel: w979 -> [w1165]
      tunnel: [w1165] -> w1024
      tunnel: w1024 -> [w1166]
      frame #0 {
        n522 = call "Wait3"("Count(Ticks)"="BD 2 Delay (Ticks)") -> ()  [unwired: 1 out]
      }
      frame #1 {
        # "switch frequency"
        n523 = xnode "FPGA I/O Node"("Connector1/DIO37"=w1166) -> ()  [unwired: 1 in, 1 out]
      }
    }
    n524 = xnode ("FIFO Read")("Timeout"=-1, "FIFO In"=w1021) -> ("Element"=w1016:u16, "FIFO Out"=w1020:refnum<k21>)  [unwired: 1 out]
    n525 = xnode ("FIFO Read")("Timeout"=-1, "FIFO In"=w1020) -> ("Element"=w1015:u16)  [unwired: 2 out]
    n526 = node-c288() -> (w1018:T7)  [unwired: 1 in]
    n527 = timed-loop "Convert amplitude words to bits" {
      timing: w1018 -> [_]
      timing-out: [_] -> w1017
      tunnel: w1016 -> [w1085]
      tunnel: w1015 -> [w1084]
      tunnel: [w1061] -> w1014
      tunnel: [w1060] -> w1013
      tunnel: [w1059] -> w1012
      tunnel: [w1058] -> w1011
      tunnel: [w1057] -> w1010
      tunnel: [w1056] -> w1009
      tunnel: [w1055] -> w1008
      tunnel: [w1054] -> w1007
      tunnel: [w1053] -> w1006
      tunnel: [w1052] -> w1005
      tunnel: [w1051] -> w1004
      tunnel: [w1050] -> w1003
      tunnel: [w1049] -> w1002
      tunnel: [w1048] -> w1001
      tunnel: [w1047] -> w1000
      tunnel: [w1046] -> w999
      tunnel: [w1045] -> w998
      tunnel: [w1044] -> w997
      tunnel: [w1043] -> w996
      tunnel: [w1042] -> w995
      tunnel: [w1041] -> w994
      tunnel: [w1040] -> w993
      tunnel: [w1039] -> w992
      tunnel: [w1038] -> w991
      tunnel: [w1037] -> w990
      tunnel: [w1036] -> w989
      tunnel: [w1035] -> w988
      tunnel: [w1034] -> w987
      tunnel: [w1033] -> w986
      tunnel: [w1032] -> w985
      tunnel: [w1031] -> w984
      tunnel: [w1030] -> w983
      stop <- TRUE stop-if-true
      # "Board 1 Data"
      # "Board 2 Data"
      # "Board 1 Data"
      # "Board 2 Data"
      n528 = Split Number(x=w1085) -> (hi(x)=w1083:u8, lo(x)=w1063:u8)
      n529 = Split Number(x=w1084) -> (hi(x)=w1082:u8, lo(x)=w1062:u8)
      n530 = Number To Boolean Array(number=w1083) -> (Boolean array=w1103:bool[])
      n531 = Number To Boolean Array(number=w1082) -> (Boolean array=w1094:bool[])
      n532 = Index Array(array=w1103, index=7) -> (element=w1061:bool)
      n533 = Index Array(array=w1103, index=6) -> (element=w1060:bool)
      n534 = Index Array(array=w1103, index=5) -> (element=w1059:bool)
      n535 = Index Array(array=w1103, index=4) -> (element=w1058:bool)
      n536 = Index Array(array=w1103, index=3) -> (element=w1057:bool)
      n537 = Index Array(array=w1103, index=2) -> (element=w1056:bool)
      n538 = Index Array(array=w1103, index=1) -> (element=w1055:bool)
      n539 = Index Array(array=w1103, index=0) -> (element=w1054:bool)
      n540 = Index Array(array=w1094, index=7) -> (element=w1053:bool)
      n541 = Index Array(array=w1094, index=6) -> (element=w1052:bool)
      n542 = Index Array(array=w1094, index=5) -> (element=w1051:bool)
      n543 = Index Array(array=w1094, index=4) -> (element=w1050:bool)
      n544 = Index Array(array=w1094, index=3) -> (element=w1049:bool)
      n545 = Index Array(array=w1094, index=2) -> (element=w1048:bool)
      n546 = Index Array(array=w1094, index=1) -> (element=w1047:bool)
      n547 = Index Array(array=w1094, index=0) -> (element=w1046:bool)
      n548 = Number To Boolean Array(number=w1063) -> (Boolean array=w1081:bool[])
      n549 = Number To Boolean Array(number=w1062) -> (Boolean array=w1072:bool[])
      n550 = Index Array(array=w1081, index=7) -> (element=w1045:bool)
      n551 = Index Array(array=w1081, index=6) -> (element=w1044:bool)
      n552 = Index Array(array=w1081, index=5) -> (element=w1043:bool)
      n553 = Index Array(array=w1081, index=4) -> (element=w1042:bool)
      n554 = Index Array(array=w1081, index=3) -> (element=w1041:bool)
      n555 = Index Array(array=w1081, index=2) -> (element=w1040:bool)
      n556 = Index Array(array=w1081, index=1) -> (element=w1039:bool)
      n557 = Index Array(array=w1081, index=0) -> (element=w1038:bool)
      n558 = Index Array(array=w1072, index=7) -> (element=w1037:bool)
      n559 = Index Array(array=w1072, index=6) -> (element=w1036:bool)
      n560 = Index Array(array=w1072, index=5) -> (element=w1035:bool)
      n561 = Index Array(array=w1072, index=4) -> (element=w1034:bool)
      n562 = Index Array(array=w1072, index=3) -> (element=w1033:bool)
      n563 = Index Array(array=w1072, index=2) -> (element=w1032:bool)
      n564 = Index Array(array=w1072, index=1) -> (element=w1031:bool)
      n565 = Index Array(array=w1072, index=0) -> (element=w1030:bool)
    }
    n566 = node-c288(w1017) -> ()
  }
  n567 = while "APD 1 Gating" {
    shift-right: [w1170] -> _
    shift-left: w2 -> [w1175]
    shift-right: [w1169] -> _
    shift-left: w4 -> [w1167]
    stop <- FALSE stop-if-true
    n568 = flat-sequence {
      tunnel: w1175 -> [w1178]
      tunnel: [w1179] -> w1173
      tunnel: [w1178] -> w1171
      tunnel: [w1177] -> w1168
      tunnel: w1167 -> [w1177]
      tunnel: [w1182] -> w1174
      tunnel: w1173 -> [w1182]
      tunnel: [w1181] -> w1172
      tunnel: w1171 -> [w1181]
      tunnel: w1168 -> [w1180]
      tunnel: [w1200] -> w1170
      tunnel: w1174 -> [w1214]
      tunnel: w1172 -> [w1211]
      tunnel: [w1183] -> w1169
      frame #0 {
        n569 = call "Loop Timer4"("Count(Ticks)"=w1178) -> ("Tick Count(Ticks)"=w1179:u32)
      }
      frame #1 {
        # "Signal maybe then sent through \na transistor before APD"
        n570 = xnode "FPGA I/O Node"("Connector0/DIO0"=w1180) -> ()  [unwired: 1 in, 1 out]
        "APD1 int gate" <- w1180
      }
      frame #2 {
        n571 = feedback #48(TRUE) -> (w1206:bool)
        n572 = feedback-in #49(w1214) -> ()
        n573 = feedback #49(w1214) -> (w1213:u32)
        n574 = Not(x=w1206) -> (.not. x?=w1203:bool)
        n575 = feedback-in #48(w1203) -> ()
        n576 = Subtract(x=w1214, y=w1213) -> (x-y=w1212:u32)
        n577 = Select(t="APD Gate ON Count", s=w1203, f="APD Gate OFF Count") -> (s? t:f=w1208:u16)
        n578 = Subtract(x=w1212, y=w1211) -> (x-y=w1188:u32)
        n579 = Subtract(x=w1208, y=w1188) -> (x-y=w1199:u32)
        n580 = Number To Boolean Array(number=w1188) -> (Boolean array=w1189:bool[])
        n581 = Or Array Elements(Boolean array=w1189) -> (logical OR=w1187:bool)
        n582 = Boolean To (0,1)(Boolean="+ phase (APD 1 Gate)") -> (0, 1=w1197:i16)
        n583 = Boolean To (0,1)(Boolean=w1187) -> (0, 1=w1194:i16)
        n584 = Multiply(x=w1197, y="Phase count adjustment (APD 1 Gate)") -> (x*y=w1195:i16)
        n585 = To Unsigned Byte Integer(number=w1194) -> (unsigned 8bit integer=w1191:u8)
        n586 = Add(x=w1199, y=w1195) -> (x+y=w1200:u32)
        n587 = feedback #50(i16 0) -> (w1202:i16)
        n588 = Subtract(x=w1202, y=w1195) -> (x-y=w1201:i16)
        "APD 1 Gate Relative Phase" <- w1201
        n589 = feedback-in #50(w1201) -> ()
        n590 = feedback #51(u8 0) -> (w1192:u8)
        n591 = Add(x=w1191, y=w1192) -> (x+y=w1190:u8)
        "APD 1 Gate Late Counter" <- w1190
        n592 = feedback-in #51(w1190) -> ()
        n593 = case shown="2" "APD Gate Operating Mode" {
          tunnel: [TRUE FALSE w1217] -> w1184
          tunnel: w1206 -> [_ _ w1217]
          frame 0, Default {
          }
          frame 1 {
          }
          frame 2 {
          }
        }
        n594 = Not(x=w1184) -> (.not. x?=w1185:bool)
        n595 = Select(t=w1185, s="Invert APD Gate", f=w1184) -> (s? t:f=w1183:bool)
      }
    }
  }
  n596 = while "APD 2 Gating" {
    shift-right: [w1221] -> _
    shift-left: w2 -> [w1226]
    shift-right: [w1220] -> _
    shift-left: w4 -> [w1218]
    stop <- FALSE stop-if-true
    n597 = flat-sequence {
      tunnel: w1226 -> [w1229]
      tunnel: [w1230] -> w1224
      tunnel: [w1229] -> w1222
      tunnel: [w1228] -> w1219
      tunnel: w1218 -> [w1228]
      tunnel: [w1233] -> w1225
      tunnel: w1224 -> [w1233]
      tunnel: [w1232] -> w1223
      tunnel: w1222 -> [w1232]
      tunnel: w1219 -> [w1231]
      tunnel: [w1255] -> w1221
      tunnel: w1225 -> [w1265]
      tunnel: w1223 -> [w1263]
      tunnel: [w1234] -> w1220
      frame #0 {
        n598 = call "Loop Timer3"("Count(Ticks)"=w1229) -> ("Tick Count(Ticks)"=w1230:u32)
      }
      frame #1 {
        # "Signal maybe then sent through \na transistor before APD"
        n599 = xnode "FPGA I/O Node"("Connector0/DIO1"=w1231) -> ()  [unwired: 1 in, 1 out]
        "APD2 int gate" <- w1231
      }
      frame #2 {
        n600 = local read "APD Gate ON Count"() -> (w1248:u16)
        n601 = local read "APD Gate OFF Count"() -> (w1247:u16)
        n602 = feedback #52(TRUE) -> (w1260:bool)
        n603 = feedback-in #53(w1265) -> ()
        n604 = feedback #53(w1265) -> (w1249:u32)
        n605 = Not(x=w1260) -> (.not. x?=w1258:bool)
        n606 = feedback-in #52(w1258) -> ()
        n607 = Subtract(x=w1265, y=w1249) -> (x-y=w1264:u32)
        n608 = Select(t=w1248, s=w1258, f=w1247) -> (s? t:f=w1262:u16)
        n609 = Subtract(x=w1264, y=w1263) -> (x-y=w1240:u32)
        n610 = Subtract(x=w1262, y=w1240) -> (x-y=w1254:u32)
        n611 = Number To Boolean Array(number=w1240) -> (Boolean array=w1239:bool[])
        n612 = Or Array Elements(Boolean array=w1239) -> (logical OR=w1238:bool)
        n613 = Boolean To (0,1)(Boolean="+ phase (APD 2 Gate)") -> (0, 1=w1252:i16)
        n614 = Multiply(x=w1252, y="Phase count adjustment (APD 2 Gate)") -> (x*y=w1250:i16)
        n615 = Boolean To (0,1)(Boolean=w1238) -> (0, 1=w1245:i16)
        n616 = Add(x=w1254, y=w1250) -> (x+y=w1255:u32)
        n617 = To Unsigned Byte Integer(number=w1245) -> (unsigned 8bit integer=w1242:u8)
        n618 = feedback #54(i16 0) -> (w1257:i16)
        n619 = Subtract(x=w1257, y=w1250) -> (x-y=w1256:i16)
        "APD 2 Gate Relative Phase" <- w1256
        n620 = feedback-in #54(w1256) -> ()
        n621 = feedback #55(u8 0) -> (w1243:u8)
        n622 = Add(x=w1242, y=w1243) -> (x+y=w1241:u8)
        "APD 2 Gate Late Counter" <- w1241
        n623 = feedback-in #55(w1241) -> ()
        n624 = local read "APD Gate Operating Mode"() -> (w1246:u8)
        n625 = case shown="2" w1246 {
          tunnel: [TRUE FALSE w1268] -> w1235
          tunnel: w1260 -> [_ _ w1268]
          frame 0, Default {
          }
          frame 1 {
          }
          frame 2 {
          }
        }
        n626 = local read "Invert APD Gate"() -> (w1237:bool)
        n627 = Not(x=w1235) -> (.not. x?=w1236:bool)
        n628 = Select(t=w1236, s=w1237, f=w1235) -> (s? t:f=w1234:bool)
      }
    }
  }
  n629 = while "532 nm green fluorescent laser interlacing (DO to IA 532 nm AOM ME amp)." {
    shift-right: [w1272] -> _
    shift-left: w2 -> [w1277]
    shift-right: [w1271] -> _
    shift-left: w3 -> [w1269]
    stop <- FALSE stop-if-true
    n630 = flat-sequence {
      tunnel: w1277 -> [w1280]
      tunnel: [w1279] -> w1275
      tunnel: [w1280] -> w1273
      tunnel: [w1281] -> w1270
      tunnel: w1269 -> [w1281]
      tunnel: [w1284] -> w1276
      tunnel: w1275 -> [w1284]
      tunnel: [w1283] -> w1274
      tunnel: w1273 -> [w1283]
      tunnel: w1270 -> [w1282]
      tunnel: [w1293] -> w1272
      tunnel: w1276 -> [w1313]
      tunnel: w1274 -> [w1310]
      tunnel: [w1302] -> w1271
      frame #0 {
        n631 = call "Loop Timer9"("Count(Ticks)"=w1280) -> ("Tick Count(Ticks)"=w1279:u32)
      }
      frame #1 {
        # "Then to PRL 440 amp\nOR to RF synth board FSK in"
        n632 = xnode "FPGA I/O Node"("Connector1/DIO39"=w1282) -> ()  [unwired: 1 in, 1 out]
      }
      frame #2 {
        n633 = feedback-in #56(w1313) -> ()
        n634 = feedback #56(w1313) -> (w1312:u32)
        n635 = Subtract(x=w1313, y=w1312) -> (x-y=w1311:u32)
        n636 = Subtract(x=w1311, y=w1310) -> (x-y=w1286:u32)
        n637 = Number To Boolean Array(number=w1286) -> (Boolean array=w1287:bool[])
        n638 = Or Array Elements(Boolean array=w1287) -> (logical OR=w1285:bool)
        n639 = Boolean To (0,1)(Boolean="+ phase (GI)") -> (0, 1=w1298:i16)
        n640 = Multiply(x=w1298, y="Phase count adjustment (GI)") -> (x*y=w1295:i16)
        n641 = Boolean To (0,1)(Boolean=w1285) -> (0, 1=w1292:i16)
        n642 = To Unsigned Byte Integer(number=w1292) -> (unsigned 8bit integer=w1289:u8)
        n643 = feedback #57(i16 0) -> (w1296:i16)
        n644 = feedback #58(u8 0) -> (w1290:u8)
        n645 = Add(x=w1289, y=w1290) -> (x+y=w1288:u8)
        "GI Late Counter" <- w1288
        n646 = feedback-in #58(w1288) -> ()
        n647 = Subtract(x=w1296, y=w1295) -> (x-y=w1294:i16)
        "GI Relative phase" <- w1294
        n648 = feedback-in #57(w1294) -> ()
        n649 = feedback #59(TRUE) -> (w1305:bool)
        n650 = case shown="2" "Operating Mode" {
          tunnel: [TRUE FALSE w1319] -> w1302
          tunnel: w1305 -> [_ _ w1316]
          frame 0, Default {
          }
          frame 1 {
          }
          frame 2 {
            n651 = Not(x=w1316) -> (.not. x?=w1318:bool)
            n652 = Select(t=w1318, s="Invert GI", f=w1316) -> (s? t:f=w1319:bool)
          }
        }
        n653 = Not(x=w1305) -> (.not. x?=w1301:bool)
        n654 = Select(t="Green interlace ON count", s=w1301, f="Green interlace OFF count") -> (s? t:f=w1307:u16)
        n655 = Subtract(x=w1307, y=w1286) -> (x-y=w1299:u32)
        n656 = Add(x=w1299, y=w1295) -> (x+y=w1293:u32)
        n657 = feedback-in #59(w1301) -> ()
      }
    }
  }
  n658 = while "Green excitation laser feedback measurement" {
    shift-right: [w1320] -> _
    shift-left: w2 -> [w1325]
    stop <- FALSE stop-if-true
    n659 = flat-sequence {
      tunnel: w1325 -> [w1327]
      tunnel: [w1328] -> w1323
      tunnel: [w1327] -> w1321
      tunnel: [w1335] -> w1324
      tunnel: w1323 -> [w1335]
      tunnel: [w1334] -> w1322
      tunnel: w1321 -> [w1334]
      tunnel: [w1347] -> w1320
      tunnel: w1324 -> [w1358]
      tunnel: w1322 -> [w1355]
      frame #0 {
        n660 = call "Loop Timer6"("Count(Ticks)"=w1327) -> ("Tick Count(Ticks)"=w1328:u32)
      }
      frame #1 {
        n661 = xnode "FPGA I/O Node"("Connector1/DIO35"=TRUE) -> ("Chassis2/Mod2/AI0"=w1333:i16, "Chassis2/Mod2/AI1"=w1332:i16, "Chassis2/Mod2/AI2"=w1329:i16)  [unwired: 4 in, 4 out]
        "Green FB Sum" <- w1329
        n662 = Bundle("Chassis2/Mod2/AI0"=w1333, "Chassis2/Mod2/AI1"=w1332, "Chassis2/Mod2/AI2"=w1329) -> (→"Green FB Signals":T10)  [unwired: 1 out]
      }
      frame #2 {
        n663 = feedback-in #60(w1358) -> ()
        n664 = feedback #60(w1358) -> (w1357:u32)
        n665 = Subtract(x=w1358, y=w1357) -> (x-y=w1356:u32)
        n666 = xnode "FPGA I/O Node"("Connector1/DIO35"=FALSE) -> ()  [unwired: 1 in, 1 out]
        n667 = Subtract(x=w1356, y=w1355) -> (x-y=w1337:u32)
        n668 = Subtract(x="Green FB Count", y=w1337) -> (x-y=w1351:u32)
        n669 = Number To Boolean Array(number=w1337) -> (Boolean array=w1338:bool[])
        n670 = Or Array Elements(Boolean array=w1338) -> (logical OR=w1336:bool)
        "Green FB Late?" <- w1336
        n671 = Boolean To (0,1)(Boolean="+ phase (Green FB)") -> (0, 1=w1349:i16)
        n672 = Boolean To (0,1)(Boolean=w1336) -> (0, 1=w1343:i16)
        n673 = Multiply(x=w1349, y="Phase count adjustment (Green FB)") -> (x*y=w1344:i16)
        n674 = Add(x=w1351, y=w1344) -> (x+y=w1347:u32)
        n675 = To Unsigned Word Integer(number=w1343) -> (unsigned 16bit integer=w1340:u16)
        n676 = feedback #61(i16 0) -> (w1346:i16)
        n677 = Subtract(x=w1346, y=w1344) -> (x-y=w1345:i16)
        "Green FB Relative Phase" <- w1345
        n678 = feedback-in #61(w1345) -> ()
        n679 = feedback #62(u16 0) -> (w1341:u16)
        n680 = Add(x=w1340, y=w1341) -> (x+y=w1339:u16)
        "Green Late Counter" <- w1339
        n681 = feedback-in #62(w1339) -> ()
      }
    }
  }
  n682 = while "Control APD data integration - stream to host" {
    shift-right: [w1361] -> _
    shift-left: w5 -> [w1366]
    stop <- FALSE stop-if-true
    n683 = flat-sequence {
      tunnel: w1366 -> [w1368]
      tunnel: [w1369] -> w1364
      tunnel: [w1368] -> w1362
      tunnel: [w1377] -> w1365
      tunnel: w1364 -> [w1377]
      tunnel: [w1376] -> w1363
      tunnel: w1362 -> [w1376]
      tunnel: [w1375] -> w1360
      tunnel: [w1374] -> w1359
      tunnel: [w1411] -> w1361
      tunnel: w1365 -> [w1423]
      tunnel: w1363 -> [w1420]
      tunnel: w1360 -> [w1404]
      tunnel: w1359 -> [w1403]
      frame #0 {
        n684 = call "Loop Timer4"("Count(Ticks)"=w1368) -> ("Tick Count(Ticks)"=w1369:u32)
      }
      frame #1 {
        n685 = flat-sequence {
          tunnel: [w1379] -> w1373
          tunnel: w1373 -> [w1381]
          tunnel: [w1383] -> w1372
          tunnel: [w1382] -> w1371
          tunnel: [w1381] -> w1370
          tunnel: [w1389] -> w1374
          tunnel: [w1390] -> w1375
          tunnel: w1372 -> [w1390]
          tunnel: w1371 -> [w1389]
          tunnel: w1370 -> [w1388]
          frame #0 {
            # "use two separate variable so each APD won't\nhave to wait to read"
            n686 = feedback #63(FALSE) -> (w1378:bool)
            "APD1 out state" <- w1378
            "APD2 out state" <- w1378
            n687 = Not(x=w1378) -> (.not. x?=w1379:bool)
            n688 = feedback-in #63(w1379) -> ()
          }
          frame #1 {
            n689 = local read "APD 1 Counts 1"() -> (w1387:u32)
            n690 = local read "APD 1 Counts 0"() -> (w1386:u32)
            n691 = local read "APD 2 Counts 1"() -> (w1385:u32)
            n692 = local read "APD 2 Counts 0"() -> (w1384:u32)
            n693 = Select(t=w1387, s=w1381, f=w1386) -> (s? t:f=w1383:u32)
            n694 = Select(t=w1385, s=w1381, f=w1384) -> (s? t:f=w1382:u32)
          }
          frame #2 {
            n695 = case shown="True" w1388 {
              frame False {
                w1391 = u32 0 ("APD 1 Counts 0")
                n696 = local write "APD 1 Counts 0"(w1391) -> ()
                n697 = local write "APD 2 Counts 0"(w1391) -> ()
              }
              frame True {
                w1392 = u32 0 ("APD 1 Counts 1")
                n698 = local write "APD 1 Counts 1"(w1392) -> ()
                n699 = local write "APD 2 Counts 1"(w1392) -> ()
              }
            }
          }
        }
      }
      frame #2 {
        n700 = feedback-in #64(w1423) -> ()
        n701 = feedback #64(w1423) -> (w1422:u32)
        n702 = Subtract(x=w1423, y=w1422) -> (x-y=w1421:u32)
        n703 = Subtract(x=w1421, y=w1420) -> (x-y=w1396:u32)
        n704 = case shown="True" "APD to FIFO" {
          tunnel: w1404 -> [_ w1426]
          tunnel: w1403 -> [_ w1424]
          frame False {
          }
          frame True {
            n705 = flat-sequence {
              tunnel: 0 ("Timeout") -> [w1428]
              tunnel: w1426 -> [w1429]
              tunnel: [w1428] -> w1425
              tunnel: w1425 -> [w1431]
              tunnel: w1424 -> [w1430]
              frame #0 {
                n706 = xnode ("FIFO Write")("Element"=w1429, "Timeout"=w1428) -> ()  [unwired: 1 in, 2 out]
              }
              frame #1 {
                n707 = xnode ("FIFO Write")("Element"=w1430, "Timeout"=w1431) -> ()  [unwired: 1 in, 2 out]
              }
            }
          }
        }
        n708 = Subtract(x="APD Acq Rate Count", y=w1396) -> (x-y=w1412:u32)
        n709 = Number To Boolean Array(number=w1396) -> (Boolean array=w1397:bool[])
        n710 = Or Array Elements(Boolean array=w1397) -> (logical OR=w1395:bool)
        "APD Acq Late?" <- w1395
        n711 = Boolean To (0,1)(Boolean=w1395) -> (0, 1=w1402:i16)
        n712 = To Unsigned Word Integer(number=w1402) -> (unsigned 16bit integer=w1399:u16)
        n713 = Boolean To (0,1)(Boolean="+ phase (APD Acq)") -> (0, 1=w1408:i16)
        n714 = feedback #65(u16 0) -> (w1400:u16)
        n715 = Add(x=w1399, y=w1400) -> (x+y=w1398:u16)
        "APD Acq Late Counter" <- w1398
        n716 = feedback-in #65(w1398) -> ()
        n717 = Multiply(x=w1408, y="Phase Count Adjustment (APD Acq)") -> (x*y=w1405:i16)
        n718 = Add(x=w1412, y=w1405) -> (x+y=w1411:u32)
        n719 = feedback #66(i16 0) -> (w1410:i16)
        n720 = Subtract(x=w1410, y=w1405) -> (x-y=w1407:i16)
        "APD Acq Relative Phase" <- w1407
        n721 = feedback-in #66(w1407) -> ()
        n722 = To Word Integer(number=w1404) -> (16bit integer=w1413:i16)
        n723 = To Word Integer(number=w1403) -> (16bit integer=w1414:i16)
        n724 = Multiply(x="APD 1 AO scale factor", y=w1413) -> (x*y=w1394:i16)
        n725 = Multiply(x="APD 2 AO scale factor", y=w1414) -> (x*y=w1393:i16)
        n726 = xnode "FPGA I/O Node"("Connector0/AO6"=w1394, "Connector0/AO7"=w1393) -> ()  [unwired: 2 in, 2 out]
      }
    }
  }
  n727 = disable-structure shown="Disabled" {
    disable-tunnel: w2 -> [w1432 _]
    frame Disabled {
      n728 = while "APD 3 Counter" {
        tunnel: w1432 -> [_]
        stop <- FALSE stop-if-true
        n729 = flat-sequence {
          frame #0 {
            n730 = xnode "FPGA I/O Method Node"("FPGA I/O In"=refnum<k21> "Connector0/DIO12" ("APD 2 DO"), "Timeout"=-1) -> ()  [unwired: 2 out]
          }
          frame #1 {
            n731 = local read "APD3 int gate"() -> (w1436:bool)
            n732 = case shown="True" w1436 {
              frame False {
              }
              frame True {
                n733 = local read item#-1() -> (w1437)
                n734 = case shown="True" w1437 {
                  frame False {
                    n735 = local read "APD 3 Counts 0"() -> (w1439:u32)
                    n736 = Increment(x=w1439) -> (x+1=→"APD 3 Counts 0":u32)
                  }
                  frame True {
                    n737 = local read "APD 3 Counts 1"() -> (w1441:u32)
                    n738 = Increment(x=w1441) -> (x+1=→"APD 3 Counts 1":u32)
                  }
                }
              }
            }
          }
        }
      }
    }
    frame Enabled {
    }
  }
  n739 = disable-structure shown="Disabled" {
    disable-tunnel: w2 -> [w1443 _]
    disable-tunnel: w4 -> [w1442 _]
    frame Disabled {
      n740 = while "APD 3 Gating" {
        shift-right: [w1447] -> _
        shift-left: w1443 -> [w1452]
        shift-right: [w1446] -> _
        shift-left: w1442 -> [w1444]
        stop <- FALSE stop-if-true
        n741 = flat-sequence {
          tunnel: w1452 -> [w1455]
          tunnel: [w1454] -> w1450
          tunnel: [w1455] -> w1448
          tunnel: [w1456] -> w1445
          tunnel: w1444 -> [w1456]
          tunnel: [w1459] -> w1451
          tunnel: w1450 -> [w1459]
          tunnel: [w1458] -> w1449
          tunnel: w1448 -> [w1458]
          tunnel: w1445 -> [w1457]
          tunnel: [w1480] -> w1447
          tunnel: w1451 -> [w1491]
          tunnel: w1449 -> [w1488]
          tunnel: [w1460] -> w1446
          frame #0 {
            n742 = call "Loop Timer5"("Count(Ticks)"=w1455) -> ("Tick Count(Ticks)"=w1454:u32)
          }
          frame #1 {
            # "Signal maybe then sent through \na transistor before APD"
            n743 = xnode "FPGA I/O Node"("Connector0/DIO2"=w1457) -> ()  [unwired: 1 in, 1 out]
            "APD3 int gate" <- w1457
          }
          frame #2 {
            n744 = local read "APD Gate OFF Count"() -> (w1465:u16)
            n745 = local read "APD Gate ON Count"() -> (w1466:u16)
            n746 = feedback #67(TRUE) -> (w1485:bool)
            n747 = feedback-in #68(w1491) -> ()
            n748 = feedback #68(w1491) -> (w1490:u32)
            n749 = Not(x=w1485) -> (.not. x?=w1483:bool)
            n750 = feedback-in #67(w1483) -> ()
            n751 = Subtract(x=w1491, y=w1490) -> (x-y=w1489:u32)
            n752 = Select(t=w1466, s=w1483, f=w1465) -> (s? t:f=w1487:u16)
            n753 = Subtract(x=w1489, y=w1488) -> (x-y=w1468:u32)
            n754 = Subtract(x=w1487, y=w1468) -> (x-y=w1479:u32)
            n755 = Number To Boolean Array(number=w1468) -> (Boolean array=w1469:bool[])
            n756 = Or Array Elements(Boolean array=w1469) -> (logical OR=w1467:bool)
            n757 = Boolean To (0,1)(Boolean=w1467) -> (0, 1=w1474:i16)
            n758 = Boolean To (0,1)(Boolean="+ phase (APD 3 Gate)") -> (0, 1=w1477:i16)
            n759 = To Unsigned Byte Integer(number=w1474) -> (unsigned 8bit integer=w1471:u8)
            n760 = Multiply(x=w1477, y="Phase count adjustment (APD 3 Gate)") -> (x*y=w1475:i16)
            n761 = feedback #69(u8 0) -> (w1472:u8)
            n762 = Add(x=w1471, y=w1472) -> (x+y=w1470:u8)
            "APD 3 Gate Late Counter" <- w1470
            n763 = feedback-in #69(w1470) -> ()
            n764 = Add(x=w1479, y=w1475) -> (x+y=w1480:u32)
            n765 = feedback #70(i16 0) -> (w1482:i16)
            n766 = Subtract(x=w1482, y=w1475) -> (x-y=w1481:i16)
            "APD 3 Gate Relative Phase" <- w1481
            n767 = feedback-in #70(w1481) -> ()
            n768 = local read "APD Gate Operating Mode"() -> (w1464:u8)
            n769 = case shown="2" w1464 {
              tunnel: [TRUE FALSE w1494] -> w1461
              tunnel: w1485 -> [_ _ w1494]
              frame 0, Default {
              }
              frame 1 {
              }
              frame 2 {
              }
            }
            n770 = local read "Invert APD Gate"() -> (w1463:bool)
            n771 = Not(x=w1461) -> (.not. x?=w1462:bool)
            n772 = Select(t=w1462, s=w1463, f=w1461) -> (s? t:f=w1460:bool)
          }
        }
      }
    }
    frame Enabled {
    }
  }
  n773 = disable-structure shown="Disabled" {
    disable-tunnel: w2 -> [w1497 _]
    disable-tunnel: w3 -> [w1496 _]
    frame Disabled {
      n774 = while "633 nm red  fluorescent laser interlacing (DO to IA 633 nm AOM ME amp)." {
        shift-right: [w1618] -> _
        shift-left: w1497 -> [w1623]
        shift-right: [w1617] -> _
        shift-left: w1496 -> [w1615]
        stop <- FALSE stop-if-true
        n775 = flat-sequence {
          tunnel: w1623 -> [w1626]
          tunnel: [w1625] -> w1621
          tunnel: [w1626] -> w1619
          tunnel: [w1627] -> w1616
          tunnel: w1615 -> [w1627]
          tunnel: [w1630] -> w1622
          tunnel: w1621 -> [w1630]
          tunnel: [w1629] -> w1620
          tunnel: w1619 -> [w1629]
          tunnel: w1616 -> [w1628]
          tunnel: [w1639] -> w1618
          tunnel: w1622 -> [w1659]
          tunnel: w1620 -> [w1656]
          tunnel: [w1648] -> w1617
          frame #0 {
            n776 = call "Loop Timer8"("Count(Ticks)"=w1626) -> ("Tick Count(Ticks)"=w1625:u32)
          }
          frame #1 {
            # "Then to PRL 440 amp"
            n777 = xnode "FPGA I/O Node"("Connector1/DIO32"=w1628) -> ()  [unwired: 1 in, 1 out]
          }
          frame #2 {
            n778 = feedback-in #71(w1659) -> ()
            n779 = feedback #71(w1659) -> (w1658:u32)
            n780 = Subtract(x=w1659, y=w1658) -> (x-y=w1657:u32)
            n781 = Subtract(x=w1657, y=w1656) -> (x-y=w1632:u32)
            n782 = Number To Boolean Array(number=w1632) -> (Boolean array=w1633:bool[])
            n783 = Or Array Elements(Boolean array=w1633) -> (logical OR=w1631:bool)
            n784 = Boolean To (0,1)(Boolean="+ phase (RI)") -> (0, 1=w1644:i16)
            n785 = Multiply(x=w1644, y="Phase count adjustment (RI)") -> (x*y=w1641:i16)
            n786 = Boolean To (0,1)(Boolean=w1631) -> (0, 1=w1638:i16)
            n787 = To Unsigned Byte Integer(number=w1638) -> (unsigned 8bit integer=w1635:u8)
            n788 = feedback #72(i16 0) -> (w1642:i16)
            n789 = feedback #73(u8 0) -> (w1636:u8)
            n790 = Add(x=w1635, y=w1636) -> (x+y=w1634:u8)
            "RI Late Counter" <- w1634
            n791 = feedback-in #73(w1634) -> ()
            n792 = Subtract(x=w1642, y=w1641) -> (x-y=w1640:i16)
            "RI Relative phase" <- w1640
            n793 = feedback-in #72(w1640) -> ()
            n794 = feedback #74(TRUE) -> (w1651:bool)
            n795 = case shown="2" "Red Laser Operating Mode" {
              tunnel: [TRUE FALSE w1665] -> w1648
              tunnel: w1651 -> [_ _ w1662]
              frame 0, Default {
              }
              frame 1 {
              }
              frame 2 {
                n796 = Not(x=w1662) -> (.not. x?=w1664:bool)
                n797 = Select(t=w1664, s="Invert RI", f=w1662) -> (s? t:f=w1665:bool)
              }
            }
            n798 = Not(x=w1651) -> (.not. x?=w1647:bool)
            n799 = Select(t="Red interlace ON count", s=w1647, f="Red interlace OFF count") -> (s? t:f=w1653:u16)
            n800 = Subtract(x=w1653, y=w1632) -> (x-y=w1645:u32)
            n801 = Add(x=w1645, y=w1641) -> (x+y=w1639:u32)
            n802 = feedback-in #74(w1647) -> ()
          }
        }
      }
      n803 = while "473 nm blue  fluorescent laser interlacing (DO to blue laser digital control input)." {
        shift-right: [w1514] -> _
        shift-left: w1497 -> [w1517]
        shift-right: [w1513] -> _
        shift-left: w1496 -> [w1511]
        shift-right: [w1506] -> _
        shift-left: _ -> [w1505]
        shift-right: [w1498] -> _
        shift-left: u16 0 -> [w1501]
        stop <- FALSE stop-if-true
        n804 = flat-sequence {
          tunnel: w1517 -> [w1520]
          tunnel: [w1519] -> w1516
          tunnel: [w1520] -> w1515
          tunnel: [w1523] -> w1512
          tunnel: w1511 -> [w1523]
          tunnel: w1505 -> [w1522]
          tunnel: [w1522] -> w1504
          tunnel: [w1521] -> w1502
          tunnel: w1501 -> [w1521]
          tunnel: [w1528] -> w1510
          tunnel: w1516 -> [w1528]
          tunnel: [w1527] -> w1509
          tunnel: w1515 -> [w1527]
          tunnel: w1512 -> [w1526]
          tunnel: w1504 -> [w1525]
          tunnel: [w1525] -> w1503
          tunnel: w1502 -> [w1524]
          tunnel: [w1524] -> w1500
          tunnel: [w1533] -> w1508
          tunnel: [w1532] -> w1507
          tunnel: w1509 -> [w1532]
          tunnel: w1510 -> [w1533]
          tunnel: w1503 -> [w1531]
          tunnel: w1500 -> [w1530]
          tunnel: [w1529] -> w1499
          tunnel: [w1590] -> w1514
          tunnel: w1508 -> [w1608]
          tunnel: w1507 -> [w1605]
          tunnel: [w1578] -> w1513
          tunnel: [w1576] -> w1506
          tunnel: w1499 -> [w1573]
          tunnel: [w1574] -> w1498
          frame #0 {
            n805 = call "Loop Timer7"("Count(Ticks)"=w1520) -> ("Tick Count(Ticks)"=w1519:u32)
          }
          frame #1 {
            n806 = xnode "FPGA I/O Node"("Connector1/DIO28"=w1526) -> ()  [unwired: 1 in, 1 out]
          }
          frame #2 {
            n807 = case shown="True" w1531 {
              tunnel: w1530 -> [w1534 w1536]
              tunnel: [w1534 w1535] -> w1529
              frame False {
              }
              frame True {
                n808 = flat-sequence {
                  tunnel: [w1542] -> w1539
                  tunnel: [w1541] -> w1538
                  tunnel: [w1540] -> w1537
                  tunnel: w1536 -> [w1540]
                  tunnel: w1539 -> [w1559]
                  tunnel: w1538 -> [w1556]
                  tunnel: w1537 -> [w1558]
                  tunnel: [w1557] -> w1535
                  frame #0 {
                    # "5 ns timing resolution"
                    n809 = node-c288() -> (w1545:T7)  [unwired: 1 in]
                    n810 = timed-loop {
                      timing: w1545 -> [_]
                      timing-out: [_] -> w1544
                      tunnel: "Lifetime timeout APD1" -> [w1551]
                      tunnel: [w1546] -> w1541
                      tunnel: [w1547] -> w1542
                      i -> [w1548]
                      stop <- w1550 stop-if-true
                      n811 = xnode "FPGA I/O Node"() -> ("Connector0/DIO5"=w1549:bool)  [unwired: 1 in, 1 out]
                      n812 = To Unsigned Word Integer(number=w1548) -> (unsigned 16bit integer=w1546:u16)
                      n813 = Equal?(x=w1551, y=w1546) -> (x = y?=w1547:bool)
                      n814 = Or(x=w1549, y=w1547) -> (x .or. y?=w1550:bool)
                    }
                    n815 = node-c288(w1544) -> ()
                  }
                  frame #1 {
                    n816 = Not(x=w1559) -> (.not. x?=w1560:bool)
                    n817 = case shown="True" w1560 {
                      tunnel: w1556 -> [_ w1562]
                      tunnel: w1558 -> [w1561 w1564]
                      tunnel: [w1561 w1563] -> w1557
                      frame False {
                        # "timed out, do nothing"
                      }
                      frame True {
                        # "photon detected,record time"
                        n818 = case shown="True" "Lifetime to FIFO" {
                          tunnel: w1562 -> [_ w1570]
                          tunnel: w1564 -> [w1566 w1568]
                          tunnel: [w1566 w1567] -> w1563
                          frame False {
                            # "don't record time\n(can't if doing force feedback)"
                          }
                          frame True {
                            # "number of events in fifo"
                            n819 = xnode ("FIFO Method Node")("Element"=w1570, "Timeout"=0) -> ()  [unwired: 1 in, 2 out]
                            n820 = Increment(x=w1568) -> (x+1=w1567:u16)
                          }
                        }
                        "lifetime (ticks)" <- w1562
                      }
                    }
                  }
                }
              }
            }
          }
          frame #3 {
            # "Reading fifo is tricky here since\nunknown # of events"
            # "For lifetime measurement:\nInterlacing and pulse falling"
            n821 = feedback-in #75(w1608) -> ()
            n822 = feedback #75(w1608) -> (w1607:u32)
            n823 = Subtract(x=w1608, y=w1607) -> (x-y=w1606:u32)
            n824 = Subtract(x=w1606, y=w1605) -> (x-y=w1583:u32)
            n825 = Number To Boolean Array(number=w1583) -> (Boolean array=w1584:bool[])
            n826 = Or Array Elements(Boolean array=w1584) -> (logical OR=w1582:bool)
            n827 = Boolean To (0,1)(Boolean="+ phase (BI D)") -> (0, 1=w1595:i16)
            n828 = Multiply(x=w1595, y="Phase count adjustment (BI D)") -> (x*y=w1592:i16)
            n829 = Boolean To (0,1)(Boolean=w1582) -> (0, 1=w1589:i16)
            n830 = To Unsigned Byte Integer(number=w1589) -> (unsigned 8bit integer=w1586:u8)
            n831 = feedback #76(i16 0) -> (w1593:i16)
            n832 = feedback #77(u8 0) -> (w1587:u8)
            n833 = Add(x=w1586, y=w1587) -> (x+y=w1585:u8)
            "Blue Late Counter (D)" <- w1585
            n834 = feedback-in #77(w1585) -> ()
            n835 = Subtract(x=w1593, y=w1592) -> (x-y=w1591:i16)
            "BI Relative phase (D)" <- w1591
            n836 = feedback-in #76(w1591) -> ()
            n837 = feedback #78(TRUE) -> (w1600:bool)
            n838 = case shown="2" "Blue Laser Operating Mode (D)" {
              tunnel: [TRUE FALSE w1614] -> w1578
              tunnel: w1600 -> [_ _ w1611]
              frame 0, Default {
              }
              frame 1 {
              }
              frame 2 {
                n839 = Not(x=w1611) -> (.not. x?=w1613:bool)
                n840 = Select(t=w1613, s="Invert BI (D)", f=w1611) -> (s? t:f=w1614:bool)
              }
            }
            n841 = Subtract(x=w1573, y="Lifetime events to read blue") -> (x-y=w1571:u16)
            n842 = Not(x=w1600) -> (.not. x?=w1598:bool)
            n843 = Select(t="Blue interlace ON count (D)", s=w1598, f="Blue interlace OFF count (D)") -> (s? t:f=w1602:u16)
            n844 = Subtract(x=w1602, y=w1583) -> (x-y=w1596:u32)
            n845 = Add(x=w1596, y=w1592) -> (x+y=w1590:u32)
            n846 = feedback-in #78(w1598) -> ()
            n847 = Select(t=w1571, s="Lifetime read blue fifo", f=w1573) -> (s? t:f=w1574:u16)
            "lifetime events in fifo" <- w1574
            n848 = Equal?(x="Blue Laser Operating Mode (D)", y=u8 2) -> (x = y?=w1579:bool)
            n849 = Not(x=w1578) -> (.not. x?=w1577:bool)
            n850 = And(x=w1577, y=w1579) -> (x .and. y?=w1576:bool)
          }
        }
      }
    }
    frame Enabled {
    }
  }
